vi "Autonomous Independent.vi"() -> ()   [LabVIEW 2017]
doc: "This VI is called when autonomous begins, and will automatically be terminated when autonomous ends. You can carry out timed or sensor driven robot movement independently without needing to return to the caller."
uses:
  Public/Documents/Cross The Road Electronics/Phoenix-LabVIEW/Motor Controller/Controls/CTRE_Phoenix_MotorControl_FeedbackDevice.ctl
  <vilib>/Rock Robotics/WPI/Solenoid/WPI_SolenoidValue.ctl
  Public/Documents/Cross The Road Electronics/Phoenix-LabVIEW/Motor Controller/Controls/CTRE_Phoenix_MotorControl_ControlMode.ctl
  <vilib>/Rock Robotics/WPI/Utilities/WPI_GetSetVariantRefNum.vi
  <vilib>/Rock Robotics/Network Tables/NT Read String.vi
  <vilib>/Rock Robotics/Network Tables/NT Write Numeric Array.vi
  <vilib>/Rock Robotics/WPI/Solenoid/WPI_SolenoidSetEnum.vi
  Public/Documents/Cross The Road Electronics/Phoenix-LabVIEW/Motor Controller/Get/CTRE_Phoenix_MotorController_GetSelectedSensorData.vi
  <vilib>/addons/control/pid/pid.llb/PID (DBL).vi
  Public/Documents/Cross The Road Electronics/Phoenix-LabVIEW/Motor Controller/Get/CTRE_Phoenix_MotorController_GetLimitSwitchStates.vi
  FIRST-3958-Controls-Library/NavX/navX Library v2/navX Library v2.lvlib
  <vilib>/addons/control/pid/NI_PID_pid.lvlib
panel:
  in  "Array":T1(array[cluster])=[{"Type"="Drive", "Parameter 1"=2.0, "Parameter 2"=0.0, "Parameter 3"=0.0, "Parameter 4"=0.5, "Field Angle"=FALSE}, {"Type"="Drive", "Parameter 1"=5.0, "Parameter 2"=45.0, "Parameter 3"=0.0, "Parameter 4"=0.6, "Field Angle"=TRUE}, {"Type"="Drive", "Parameter 1"=10.0, "Parameter 2"=0.0, "Parameter 3"=1.6, "Parameter 4"=0.5, "Field Angle"=FALSE}, {"Type"="Lift", "Parameter 1"=-1000.0, "Parameter 2"=0.0, "Parameter 3"=0.3, "Parameter 4"=0.5, "Field Angle"=FALSE}, {"Type"="Wait", "Parameter 1"=0.5, "Parameter 2"=0.0, "Parameter 3"=0.0, "Parameter 4"=0.0, "Field Angle"=FALSE}, {"Type"="Drive", "Parameter 1"=-4.3, "Parameter 2"=0.0, "Parameter 3"=0.0, "Parameter 4"=0.5, "Field Angle"=FALSE}, {"Type"="Turn", "Parameter 1"=0.0, "Parameter 2"=-90.0, "Parameter 3"=0.0, "Parameter 4"=0.5, "Field Angle"=TRUE}, {"Type"="Drive", "Parameter 1"=4.0, "Parameter 2"=-90.0, "Parameter 3"=0.0, "Parameter 4"=0.3, "Field Angle"=TRUE}, {"Type"="Turn", "Parameter 1"=0.0, "Parameter 2"=0.0, "Parameter 3"=0.0, "Parameter 4"=0.5, "Field Angle"=FALSE}, {"Type"="Lift", "Parameter 1"=-2170.0, "Parameter 2"=0.0, "Parameter 3"=1.5, "Parameter 4"=0.5, "Field Angle"=FALSE}, {"Type"="Intake", "Parameter 1"=1.0, "Parameter 2"=0.0, "Parameter 3"=0.0, "Parameter 4"=0.0, "Field Angle"=FALSE}, {"Type"="Grab", "Parameter 1"=1.0, "Parameter 2"=0.0, "Parameter 3"=0.0, "Parameter 4"=0.0, "Field Angle"=FALSE}, {"Type"="Drive", "Parameter 1"=3.0, "Parameter 2"=0.0, "Parameter 3"=0.5, "Parameter 4"=0.5, "Field Angle"=FALSE}, {"Type"="Grab", "Parameter 1"=0.0, "Parameter 2"=0.0, "Parameter 3"=0.0, "Parameter 4"=0.0, "Field Angle"=FALSE}, {"Type"="Intake", "Parameter 1"=0.0, "Parameter 2"=0.0, "Parameter 3"=0.0, "Parameter 4"=0.0, "Field Angle"=FALSE}, {"Type"="Drive", "Parameter 1"=-3.0, "Parameter 2"=0.0, "Parameter 3"=0.0, "Parameter 4"=0.5, "Field Angle"=FALSE}, {"Type"="Turn", "Parameter 1"=0.0, "Parameter 2"=90.0, "Parameter 3"=0.0, "Parameter 4"=0.5, "Field Angle"=TRUE}, {"Type"="Drive", "Parameter 1"=4.6, "Parameter 2"=90.0, "Parameter 3"=0.0, "Parameter 4"=0.6, "Field Angle"=TRUE}, {"Type"="Turn", "Parameter 1"=0.0, "Parameter 2"=0.0, "Parameter 3"=0.0, "Parameter 4"=0.5, "Field Angle"=FALSE}, {"Type"="Drive", "Parameter 1"=10.0, "Parameter 2"=0.0, "Parameter 3"=0.0, "Parameter 4"=0.6, "Field Angle"=FALSE}, {"Type"="Lift", "Parameter 1"=0.0, "Parameter 2"=0.0, "Parameter 3"=1.5, "Parameter 4"=0.5, "Field Angle"=FALSE}, {"Type"="Intake", "Parameter 1"=-1.0, "Parameter 2"=0.0, "Parameter 3"=0.0, "Parameter 4"=0.0, "Field Angle"=FALSE}]
  in  "stop":bool
  in  "elevator PID":T2={"proportional gain (Kc)"=0.005, "integral time (Ti, min)"=0.0, "derivative time (Td, min)"=0.0} {"derivative time (Td, min)" format="%.3f"; "integral time (Ti, min)" format="%.3f"; "proportional gain (Kc)" format="%.3f"}
  in  "elevatorPosition":dbl=1500.0 format="%.2f"
  in  "forward PID":T2={"proportional gain (Kc)"=0.001, "integral time (Ti, min)"=0.0, "derivative time (Td, min)"=0.0} {"derivative time (Td, min)" format="%.3f"; "integral time (Ti, min)" format="%.3f"; "proportional gain (Kc)" format="%.3f"}
  in  "angle PID":T2={"proportional gain (Kc)"=0.018, "integral time (Ti, min)"=0.0, "derivative time (Td, min)"=0.0} {"derivative time (Td, min)" format="%.3f"; "integral time (Ti, min)" format="%.3f"; "proportional gain (Kc)" format="%.3f"}
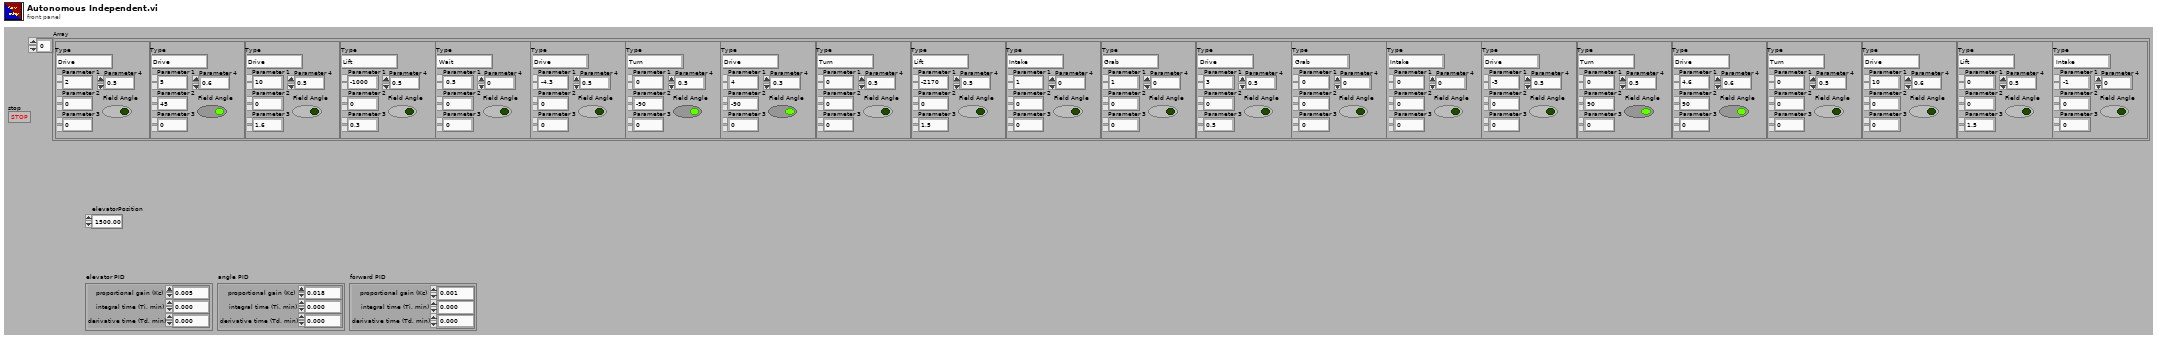
[diagram p1: front panel]
types:
  T1 = cluster{"Type":string, "Parameter 1":dbl, "Parameter 2":dbl, "Parameter 3":dbl, "Parameter 4":dbl, "Field Angle":bool}[]
  T2 = cluster{"proportional gain (Kc)":dbl, "integral time (Ti, min)":dbl, "derivative time (Td, min)":dbl}
  T3 = typedef "WPI_SolenoidValue.ctl" = enum16{"Off", "On", "Forward", "Reverse"}
  T4 = typedef "CTRE_Phoenix_MotorControl_FeedbackDevice.ctl" = i8
  T5 = typedef "WPI_JoystickDevRef.ctl" = cluster{"Device":T6}
  T6 = typedef "WPI_JoystickDeviceEnum.ctl" = enum16{"USB 0", "USB 1", "USB 2", "USB 3", "USB 4", "USB 5"}
  T7 = typedef "WPI_MotorControlDeviceRef.ctl" = cluster{"DeviceStatus":errorcluster, "Type":T8, "PWM":cluster{"PWM Channel":T9, "DeadBand":T10}, "CAN":cluster{"Device Number":u8, "SetOutput VI Ref":variant, "GetOutput VI Ref":variant, "Enable VI Ref":variant, "Disable VI Ref":variant, "Data":variant}, "Invert":bool, "DIO PWM":cluster{"PWM \"Enable\" Channel":T9, "DIOChannel":T11, "PWM Rate":dbl}}
  T8 = typedef "WPI_MotorControlType.ctl" = enum16{"PWM", "CAN", "DIO PWM"}
  T9 = typedef "FPGA_DIOPWMChannel.ctl" = enum8{"PWM 0", "PWM 1", "PWM 2", "PWM 3", "PWM 4", "PWM 5", "PWM 6", "PWM 7", "PWM 8", "PWM 9", "PWM MXP 0", "PWM MXP 1", "PWM MXP 2", "PWM MXP 3", "PWM MXP 4", "PWM MXP 5", "PWM MXP 6", "PWM MXP 7", "PWM MXP 8", "PWM MXP 9", "Invalid"}
  T10 = typedef "WPI_PWMDeadband.ctl" = cluster{"Name":string, "maxPositivePwm":i32, "minPositivePwm":i32, "centerPwm":i32, "maxNegativePwm":i32, "minNegativePwm":i32, "angularRange":u16}
  T11 = typedef "FPGA_DIOChannel.ctl" = enum8{"DIO 0", "DIO 1", "DIO 2", "DIO 3", "DIO 4", "DIO 5", "DIO 6", "DIO 7", "DIO 8", "DIO 9", "DIO MXP 0", "DIO MXP 1", "DIO MXP 2", "DIO MXP 3", "DIO MXP 4", "DIO MXP 5", "DIO MXP 6", "DIO MXP 7", "DIO MXP 8", "DIO MXP 9", "DIO MXP 10", "DIO MXP 11", "DIO MXP 12", "DIO MXP 13", "DIO MXP 14", "DIO MXP 15", "SPI Port CS1", "SPI Port CS2", "SPI Port CS3", "SPI Port MISO", "SPI Port MOSI", "Invalid"}
  T12 = typedef "WPI_SolenoidDevRef.ctl" = cluster{"DevStatus":errorcluster, "Pneumatics Control Module":u8, "Forward Solenoid Channel":T13, "Reverse Solenoid Channel":T13}
  T13 = typedef "WPI_SolenoidChannel.ctl" = enum8{"Solenoid 0", "Solenoid 1", "Solenoid 2", "Solenoid 3", "Solenoid 4", "Solenoid 5", "Solenoid 6", "Solenoid 7", "Invalid"}
  T14 = typedef "navX Library v2.lvlib/Z900_navX_DeviceTypeDef.ctl" = cluster{"Interface":cluster{"Protocol":T15, "Update Rate (4Hz-100Hz)":u8, "navX Open TypeDef":variant}, "Notify Packet":refnum<notifier>, "Loop VI Refnum":refnum<vi>, "Ready to Close Occurrence Refnum":refnum<k4>}
  T15 = typedef "navX Library v2.lvlib/Z900_navX_ProtocolTypeDef.ctl" = enum16{"SERIAL", "I2C", "SPI"}
  T16 = typedef "CTRE_Phoenix_MotorControl_ControlMode.ctl" = u16
  T17 = cluster{"Yaw":dbl, "Roll":dbl, "Pitch":dbl, "Heading":dbl, "Fused Heading":dbl}
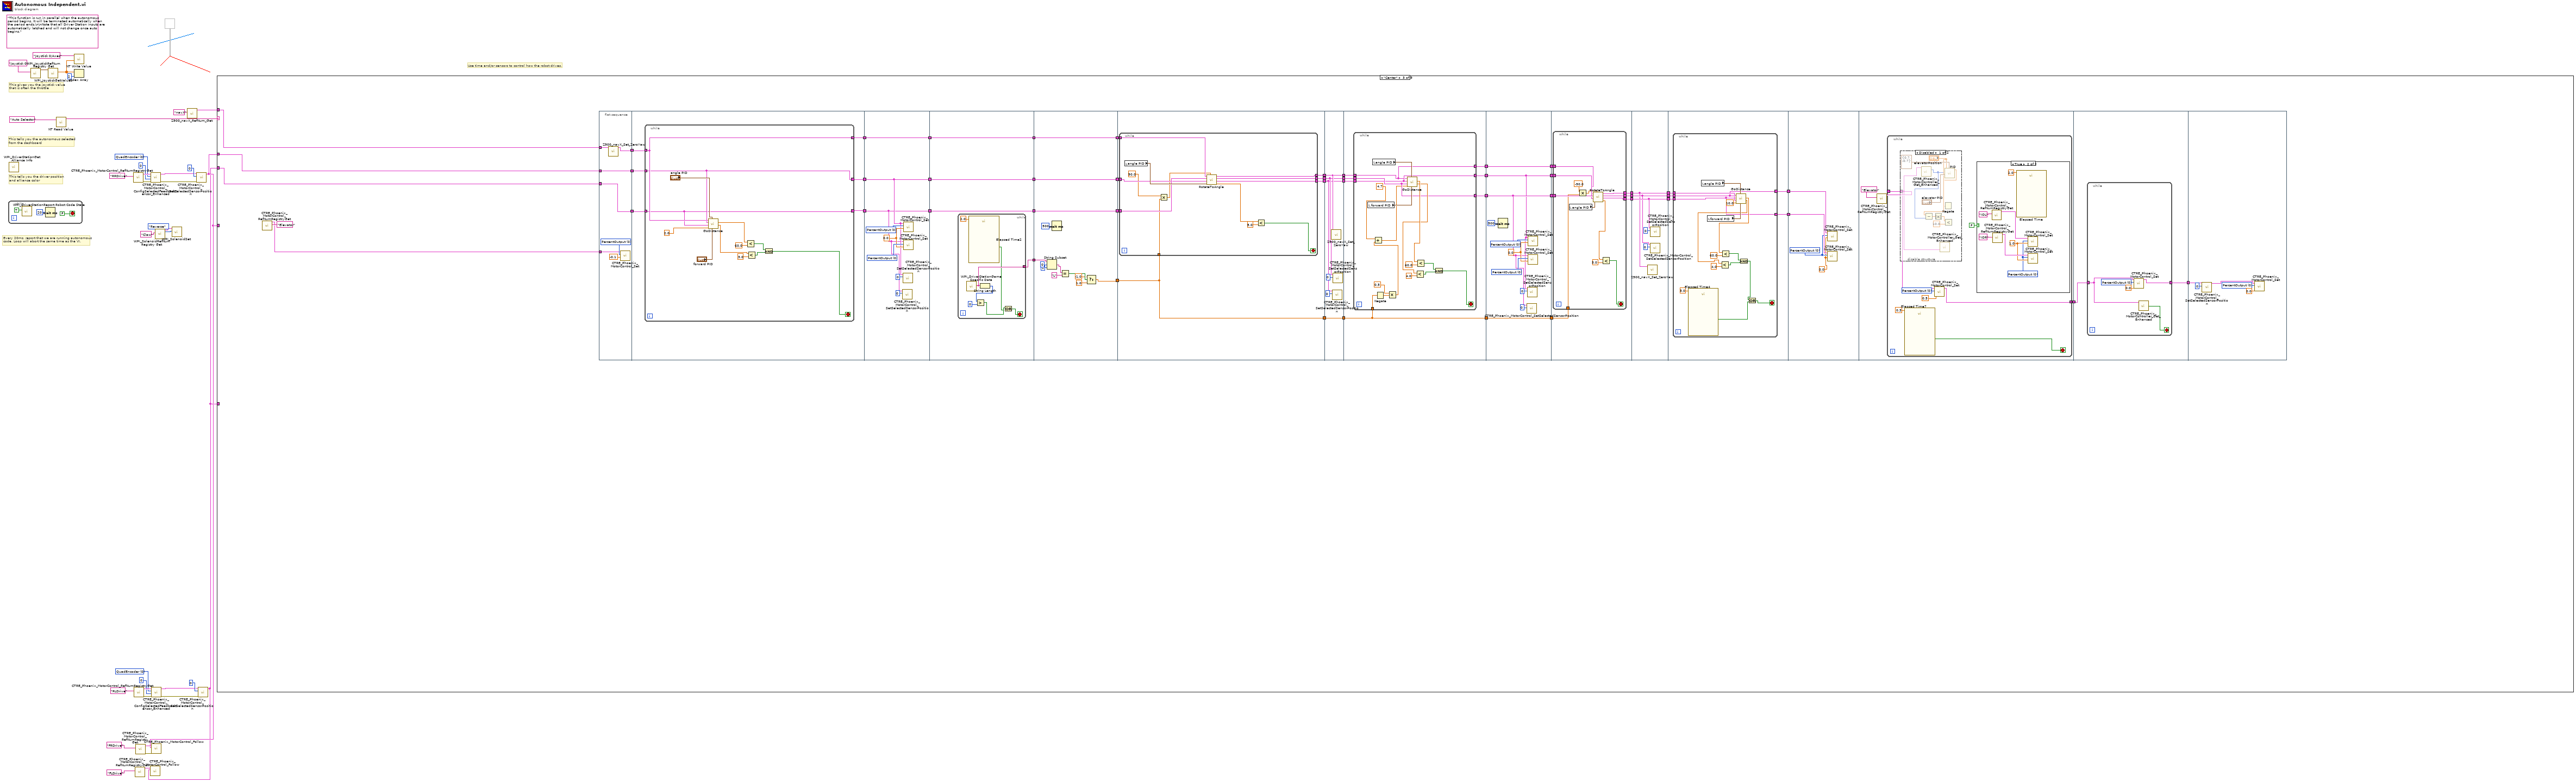
[diagram p0: block diagram]
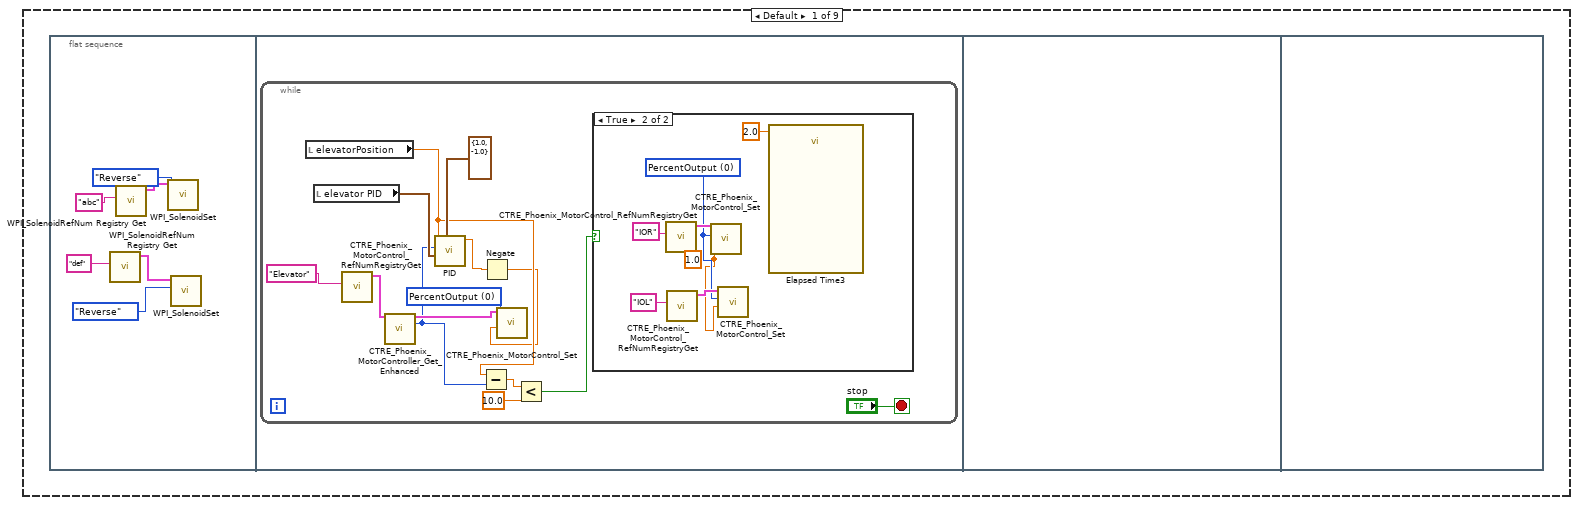
[diagram p2: hidden frame]
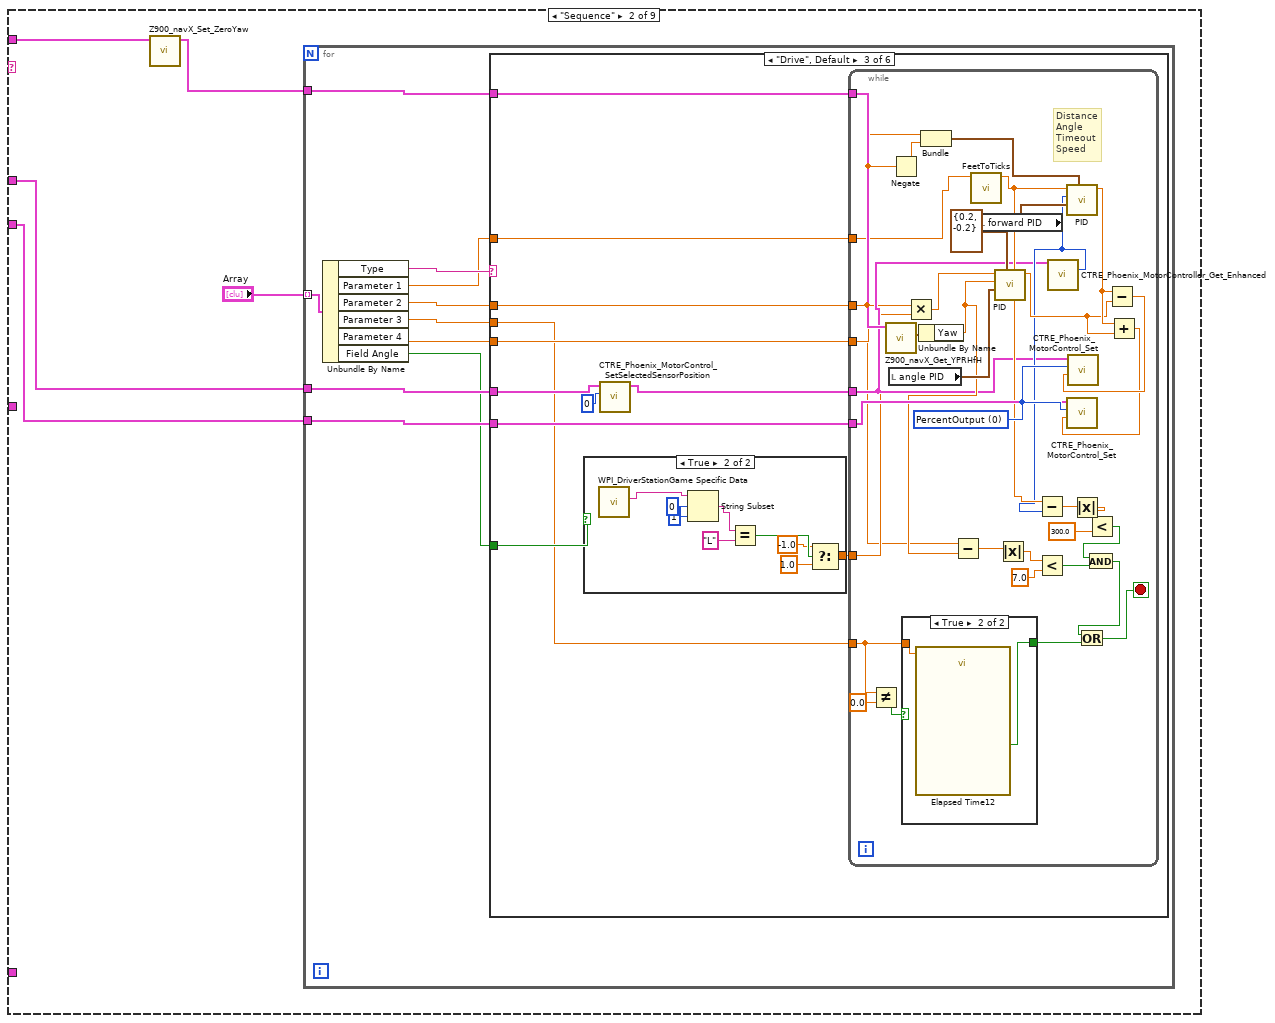
[diagram p4: hidden frame]
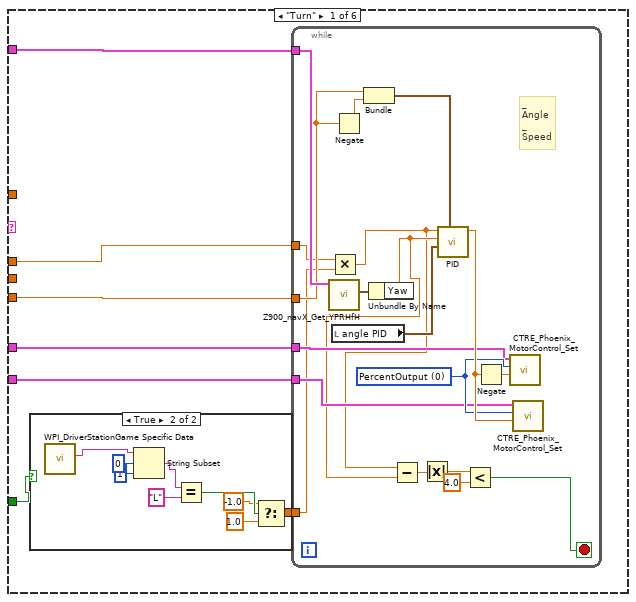
[diagram p5: hidden frame]
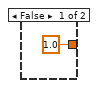
[diagram p6: hidden frame]
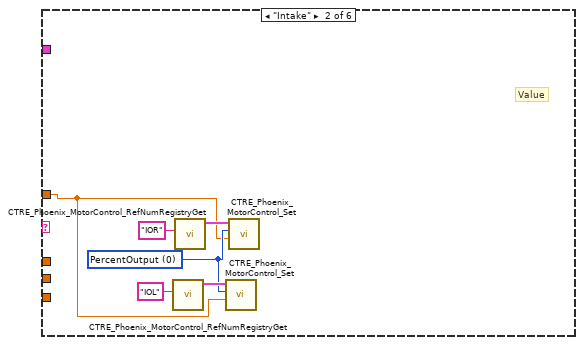
[diagram p7: hidden frame]
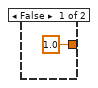
[diagram p8: hidden frame]
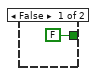
[diagram p9: hidden frame]
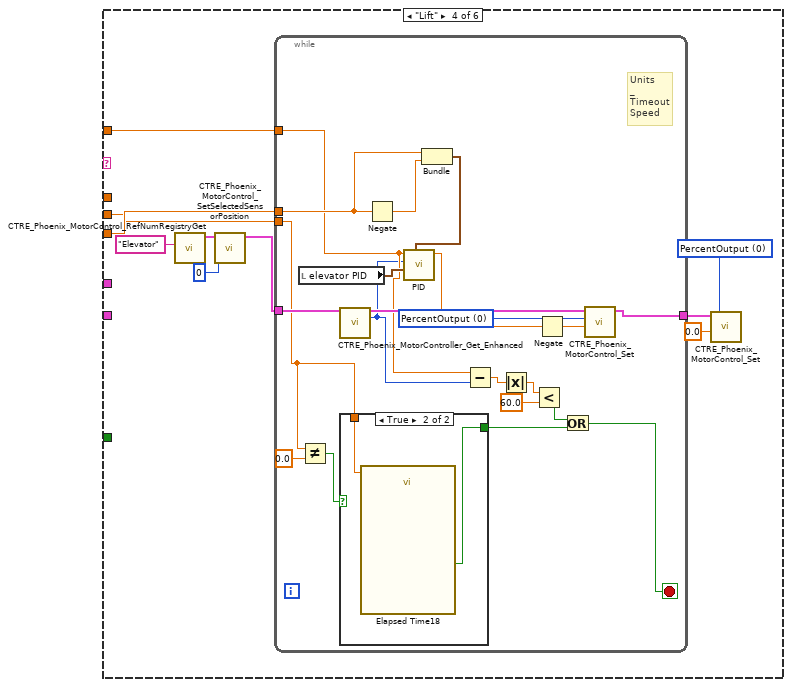
[diagram p10: hidden frame]
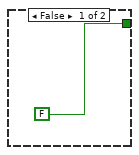
[diagram p11: hidden frame]
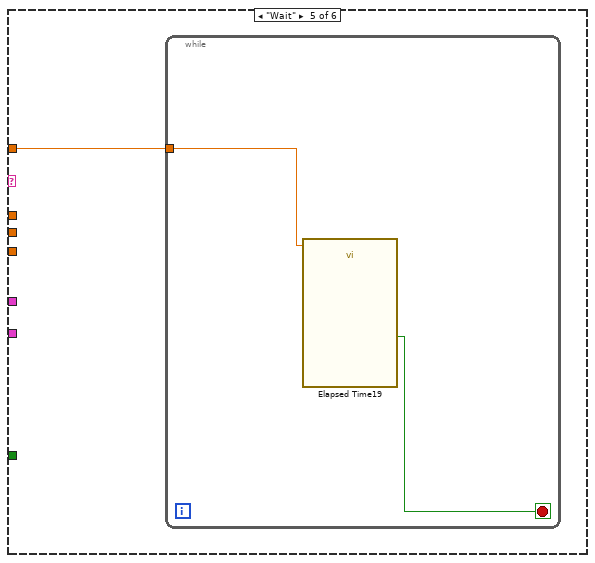
[diagram p12: hidden frame]
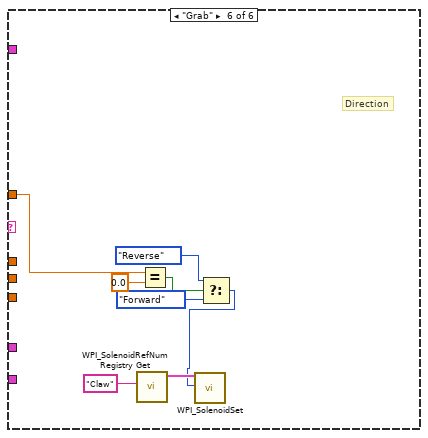
[diagram p13: hidden frame]
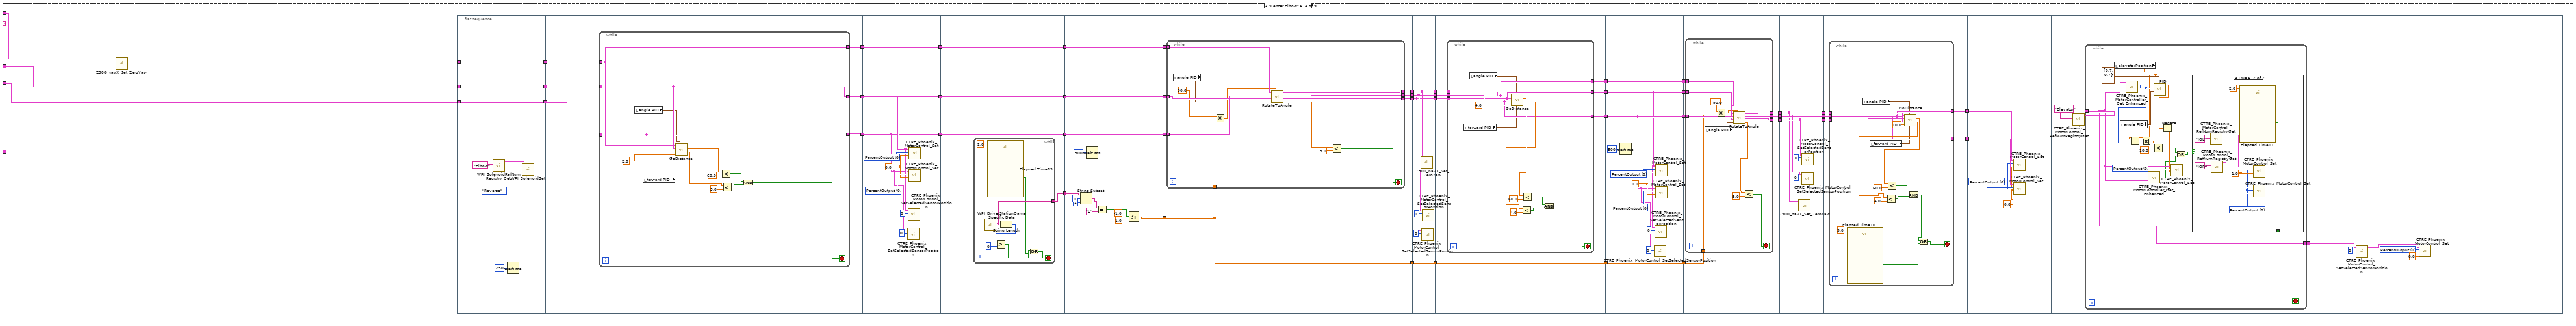
[diagram p16: hidden frame]
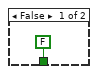
[diagram p17: hidden frame]
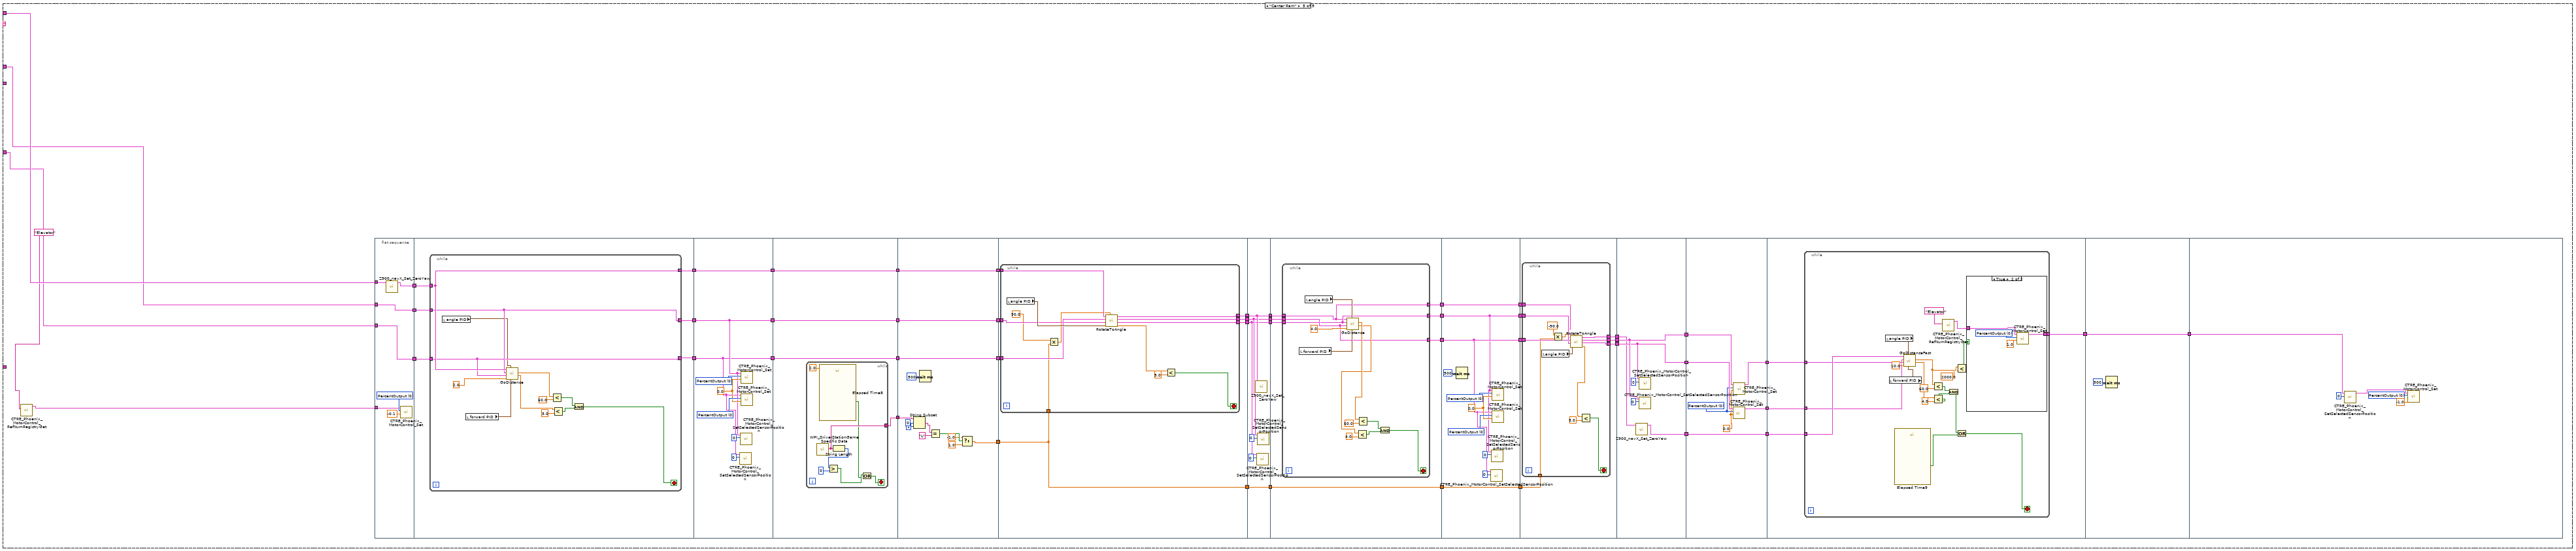
[diagram p18: hidden frame]
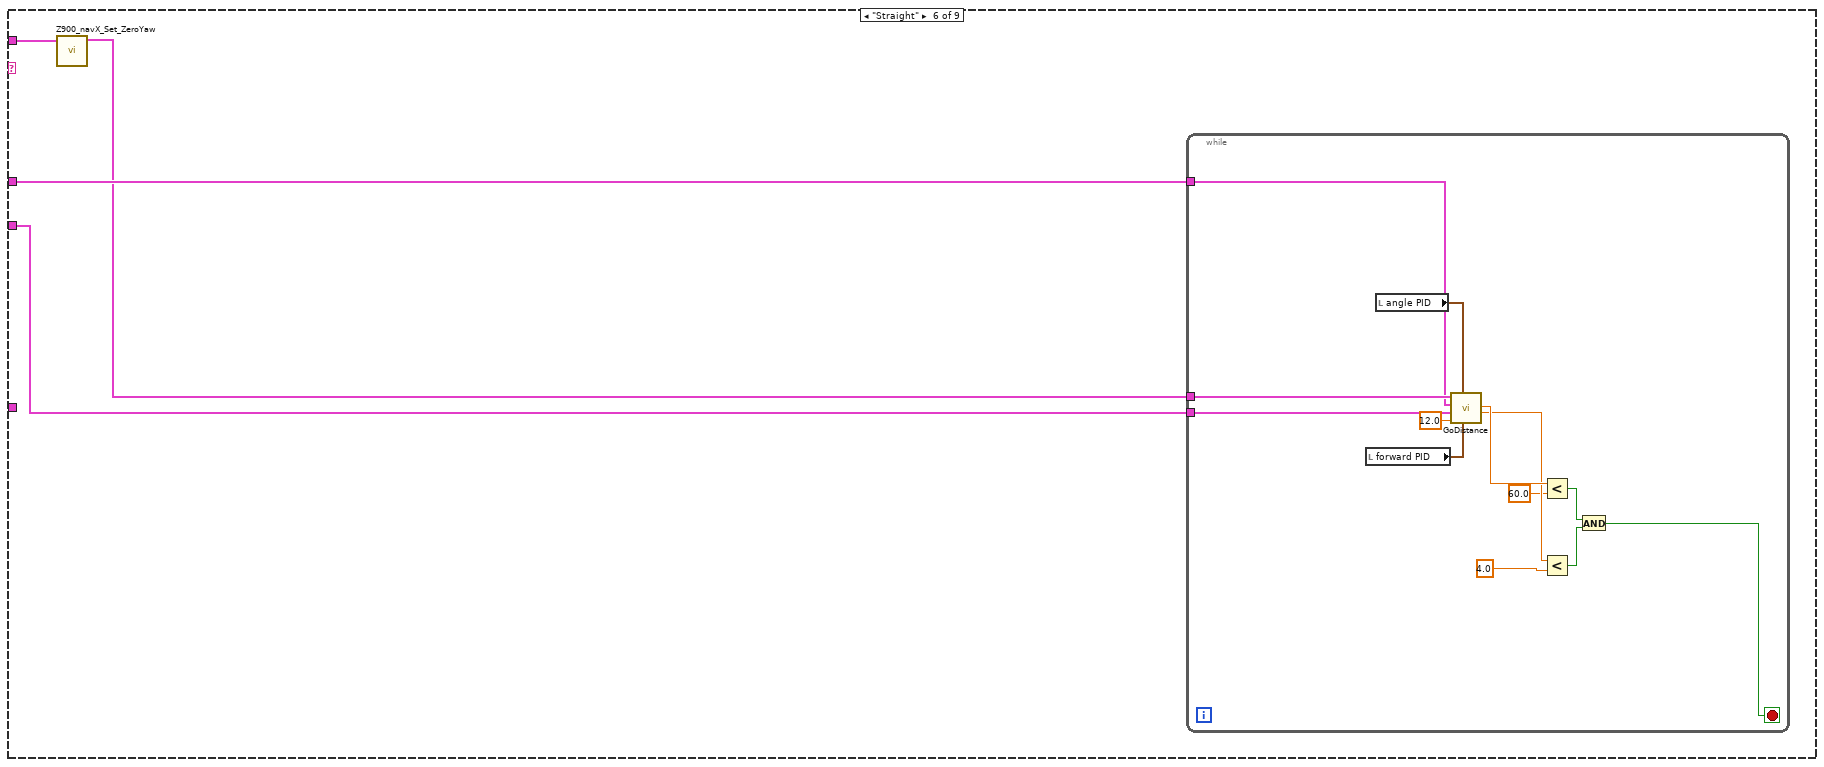
[diagram p20: hidden frame]
diagram:
  w19 = T4 0 items=["None"=-1, "QuadEncoder"=0, "Analog"=2, "Tachometer"=4, "Pulse Width Encoded Position"=8, "Sensor Sum (S0 + S1)"=9, "Sensor Difference (D0 - D1)"=10, "Remote Source 0"=11, "Remote Source 1"=12, "Software Emulated"=15] ("Feedback Device")
  w24 = T4 0 items=["None"=-1, "QuadEncoder"=0, "Analog"=2, "Tachometer"=4, "Pulse Width Encoded Position"=8, "Sensor Sum (S0 + S1)"=9, "Sensor Difference (D0 - D1)"=10, "Remote Source 0"=11, "Remote Source 1"=12, "Software Emulated"=15] ("Feedback Device")
  (unwired) "This function is run in parallel when the autonomous period begins. It will be terminated automatically when the period ends.\n\nNote that all Driver Station inputs are automatically latched and will not change once auto begins."
  # "This tells you the autonomous selected\nfrom the dashboard"
  # "Every 20ms, report that we are running autonomous\ncode. Loop will abort the same time as the VI."
  # "This gives you the joystick value\nthat is often the throttle"
  # "Use time and/or sensors to control how the robot drives."
  # "This tells you the driver position\nand alliance color"
  n1 = while {
    stop <- FALSE stop-if-true
    n2 = call <vilib>:"WPI_DriverStationReport Robot Code State.vi"("Autonomous"=TRUE) -> ()  [unwired: 10 in, 1 out]
    n3 = Wait (ms)(milliseconds to wait=u32 20) -> ()  [unwired: 1 out]
  }
  n4 = call <vilib>:"WPI_DriverStationGet Alliance Info.vi"() -> ()  [unwired: 12 out]
  n5 = call <vilib>:"WPI_JoystickRefNum Registry Get.vi"("refnum name"="Joystick 0") -> ("JoystickDevRef"=w34:T5)  [unwired: 1 in, 9 out]
  n6 = call <vilib>:"WPI_JoystickGetValues.vi"("JoystickDevRef"=w34) -> ("Axes"=w30:dbl[])  [unwired: 6 in, 4 out]
  n7 = call-poly <vilib>:"NT Read Value.vi"("Name"="Auto Selector") -> ("String"=w31:string)  [unwired: 9 in, 1 out]
  n8 = call-poly <vilib>:"NT Write Value.vi"("Numeric Array"=w30, "Name"="Joystick 0/Axes") -> ()  [unwired: 9 in, 1 out]
  n9 = Index Array(array=w30, index=2) -> ()  [unwired: 1 out]
  n10 = call "CTRE_Phoenix_MotorControl_RefNumRegistryGet.vi"("refnum name"="RRDrive") -> ("error out"=w27:errorcluster, "PhoenixMotorControlDevRef"=w26:T7)  [unwired: 9 in]
  n11 = call "CTRE_Phoenix_MotorControl_RefNumRegistryGet.vi"("refnum name"="RLDrive") -> ("error out"=w22:errorcluster, "PhoenixMotorControlDevRef"=w21:T7)  [unwired: 9 in]
  n12 = call "CTRE_Phoenix_MotorControl_RefNumRegistryGet.vi"("refnum name"="FLDrive") -> ("PhoenixMotorControlDevRef"=w10:T7)  [unwired: 9 in, 1 out]
  n13 = call "CTRE_Phoenix_MotorControl_RefNumRegistryGet.vi"("refnum name"="FRDrive") -> ("error out"=w12:errorcluster, "PhoenixMotorControlDevRef"=w11:T7)  [unwired: 9 in]
  n14 = call "CTRE_Phoenix_MotorControl_ConfigSelectedFeedbackSensor_Enhanced.vi"("error in (no error)"=w27, "pidLoopIdx"=0, "Feedback Device"=w24, "PhoenixMotorControlDevRef"=w26) -> ("error out"=w6:errorcluster, "PhoenixMotorControlDevRef"=w7:T7)  [unwired: 6 in]
  n15 = call "CTRE_Phoenix_MotorControl_ConfigSelectedFeedbackSensor_Enhanced.vi"("error in (no error)"=w22, "pidLoopIdx"=0, "Feedback Device"=w19, "PhoenixMotorControlDevRef"=w21) -> ("error out"=w4:errorcluster, "PhoenixMotorControlDevRef"=w5:T7)  [unwired: 6 in]
  n16 = call <vilib>:"WPI_SolenoidRefNum Registry Get.vi"("refnum name"="Claw") -> ("SolenoidDevRef"=w3:T12)  [unwired: 9 in, 1 out]
  n17 = call-poly <vilib>:"WPI_SolenoidSet.vi"("Value"=WPI_SolenoidValue."Reverse", "SolenoidDevRef"=w3) -> ()  [unwired: 8 in, 2 out]
  n18 = call "Z900_navX_RefNum_Get.vi"("refnum name"="navX") -> ("navX Device"=w15:T14)  [unwired: 9 in, 1 out]
  n19 = call "CTRE_Phoenix_MotorControl_SetSelectedSensorPosition.vi"("error in (no error)"=w6, "New Sensor Position"=0, "PhoenixMotorControlDevRef"=w7) -> ("PhoenixMotorControlDevRef"=w9:T7)  [unwired: 7 in, 1 out]
  n20 = call "CTRE_Phoenix_MotorControl_Follow.vi"("error in (no error)"=w12, "Master Controller to Follow"=w9, "PhoenixMotorControlDevRef"=w11) -> ()  [unwired: 7 in, 2 out]
  n21 = call "CTRE_Phoenix_MotorControl_SetSelectedSensorPosition.vi"("error in (no error)"=w4, "New Sensor Position"=0, "PhoenixMotorControlDevRef"=w5) -> ("PhoenixMotorControlDevRef"=w8:T7)  [unwired: 7 in, 1 out]
  n22 = call "CTRE_Phoenix_MotorControl_Follow.vi"("Master Controller to Follow"=w8, "PhoenixMotorControlDevRef"=w10) -> ()  [unwired: 8 in, 2 out]
  n23 = case shown="\"Center\"" w31 {
    tunnel: w9 -> [_ w67 w272 w528 w734 w959 w975 w1069 _]
    tunnel: w8 -> [_ w66 w271 w527 _ w960 w974 w1068 _]
    tunnel: w15 -> [_ w69 w275 w487 w735 w958 w976 w1070 _]
    tunnel: w9 -> [_ _ _ _ w733 _ _ _ _]
    tunnel: w8 -> [_ _ _ _ _ _ _ _ _]
    frame Default {
      n24 = flat-sequence {
        frame #0 {
          n25 = call <vilib>:"WPI_SolenoidRefNum Registry Get.vi"("refnum name"="def") -> ("SolenoidDevRef"=w42:T12)  [unwired: 9 in, 1 out]
          n26 = call <vilib>:"WPI_SolenoidRefNum Registry Get.vi"("refnum name"="abc") -> ("SolenoidDevRef"=w41:T12)  [unwired: 9 in, 1 out]
          n27 = call-poly <vilib>:"WPI_SolenoidSet.vi"("Value"=WPI_SolenoidValue."Reverse", "SolenoidDevRef"=w41) -> ()  [unwired: 8 in, 2 out]
          n28 = call-poly <vilib>:"WPI_SolenoidSet.vi"("Value"=WPI_SolenoidValue."Reverse", "SolenoidDevRef"=w42) -> ()  [unwired: 8 in, 2 out]
        }
        frame #1 {
          n29 = while {
            stop <- "stop" stop-if-true
            w54 = T16 0 items=["PercentOutput"=0, "Position"=1, "Velocity"=2, "Current"=3, "Follower"=5, "MotionProfile"=6, "MotionMagic"=7, "MotionMagicArc"=8, "MotionProfileArc"=10, "Disabled"=15] ("Control Mode")
            n30 = local read "elevatorPosition"() -> (w52:dbl)
            n31 = local read "elevator PID"() -> (w58:T2)
            n32 = call "CTRE_Phoenix_MotorControl_RefNumRegistryGet.vi"("refnum name"="Elevator") -> ("PhoenixMotorControlDevRef"=w56:T7)  [unwired: 9 in, 1 out]
            n33 = call-poly "CTRE_Phoenix_MotorController_Get_Enhanced.vi"("PhoenixMotorControlDevRef"=w56) -> ("PhoenixMotorControlDevRef"=w53:T7, "Position (Raw Sensor Units)"=w51:i32)  [unwired: 11 in, 2 out]
            n34 = call-poly <vilib>:"PID.vi"("output range"=cluster{"output high":dbl, "output low":dbl} {"output high"=1.0, "output low"=-1.0}, "PID gains"=w58, "process variable"=w51, "setpoint"=w52) -> ("output"=w48:dbl)  [unwired: 6 in, 1 out]
            n35 = Subtract(x=w52, y=w51) -> (x-y=w50:dbl)
            n36 = Negate(x=w48) -> (-x=w47:dbl)
            n37 = call "CTRE_Phoenix_MotorControl_Set.vi"("Output"=w47, "Control Mode"=w54, "PhoenixMotorControlDevRef"=w53) -> ()  [unwired: 7 in, 2 out]
            n38 = Less?(x=w50, y=10.0) -> (x < y?=w45:bool)
            n39 = case shown="True" w45 {
              frame False {
              }
              frame True {
                w60 = 1.0 ("Output")
                w61 = T16 0 items=["PercentOutput"=0, "Position"=1, "Velocity"=2, "Current"=3, "Follower"=5, "MotionProfile"=6, "MotionMagic"=7, "MotionMagicArc"=8, "MotionProfileArc"=10, "Disabled"=15] ("Control Mode")
                n40 = call "CTRE_Phoenix_MotorControl_RefNumRegistryGet.vi"("refnum name"="IOR") -> ("PhoenixMotorControlDevRef"=w62:T7)  [unwired: 9 in, 1 out]
                n41 = call "CTRE_Phoenix_MotorControl_RefNumRegistryGet.vi"("refnum name"="IOL") -> ("PhoenixMotorControlDevRef"=w63:T7)  [unwired: 9 in, 1 out]
                n42 = call "CTRE_Phoenix_MotorControl_Set.vi"("Output"=w60, "Control Mode"=w61, "PhoenixMotorControlDevRef"=w62) -> ()  [unwired: 7 in, 2 out]
                n43 = call "CTRE_Phoenix_MotorControl_Set.vi"("Output"=w60, "Control Mode"=w61, "PhoenixMotorControlDevRef"=w63) -> ()  [unwired: 7 in, 2 out]
                n44 = call "Elapsed Time3"("Time Target (s)"=2.0) -> ()  [unwired: 11 in, 8 out]
              }
            }
          }
        }
        frame #2 {
        }
        frame #3 {
        }
      }
    }
    frame "Sequence" {
      n45 = call "Z900_navX_Set_ZeroYaw.vi"("navX Device"=w69) -> ("navX Device"=w68:T14)  [unwired: 9 in, 1 out]
      n46 = for {
        tunnel: "Array" -> [w80] mode=indexing
        tunnel: w68 -> [w78]
        tunnel: w67 -> [w74]
        tunnel: w66 -> [w73]
        n47 = Unbundle By Name(w80) -> ("Type"=w79:string, "Parameter 1"=w75:dbl, "Parameter 2"=w76:dbl, "Parameter 3"=w71:dbl, "Parameter 4"=w77:dbl, "Field Angle"=w72:bool)
        n48 = case shown="\"Drive\", Default" w79 {
          tunnel: w77 -> [w85 _ w132 w188 _ _]
          tunnel: w76 -> [w87 _ w133 _ _ _]
          tunnel: w78 -> [w86 _ w131 _ _ _]
          tunnel: w75 -> [_ w117 w130 w187 w217 w227]
          tunnel: w74 -> [w84 _ w128 _ _ _]
          tunnel: w73 -> [w83 _ w129 _ _ _]
          tunnel: w72 -> [w82 _ w125 _ _ _]
          tunnel: w71 -> [_ _ w123 w186 _ _]
          frame "Turn" {
            n49 = case shown="True" w82 {
              tunnel: [1.0 ("f") w89] -> w81
              frame False {
              }
              frame True {
                n50 = call <vilib>:"WPI_DriverStationGame Specific Data.vi"() -> ("Game Specific Data"=w90:string)  [unwired: 11 in]
                n51 = String Subset(string=w90, offset (0)=0, length (rest)=1 ("length (rest)")) -> (substring=w96:string)
                n52 = Equal?(x=w96, y="L") -> (x = y?=w97:bool)
                n53 = Select(t=-1.0, s=w97, f=1.0) -> (s? t:f=w89:dbl)
              }
            }
            n54 = while {
              tunnel: w87 -> [w99]
              tunnel: w86 -> [w115]
              tunnel: w85 -> [w114]
              tunnel: w84 -> [w107]
              tunnel: w83 -> [w106]
              tunnel: w81 -> [w100]
              stop <- w101 stop-if-true
              w108 = T16 0 items=["PercentOutput"=0, "Position"=1, "Velocity"=2, "Current"=3, "Follower"=5, "MotionProfile"=6, "MotionMagic"=7, "MotionMagicArc"=8, "MotionProfileArc"=10, "Disabled"=15] ("Control Mode")
              # "_\nAngle\n_\nSpeed"
              n55 = call "Z900_navX_Get_YPRHfH.vi"("navX Device"=w115) -> ("YRPHfH"=w116:T17)  [unwired: 7 in, 3 out]
              n56 = Multiply(x=w99, y=w100) -> (x*y=w98:dbl)
              n57 = local read "angle PID"() -> (w111:T2)
              n58 = Negate(x=w114) -> (-x=w113:dbl)
              n59 = Bundle("Parameter 4"=w114, w113) -> (w112:cluster{"Parameter 4":dbl, dbl})  [unwired: 1 in]
              n60 = Unbundle By Name(w116) -> ("Yaw"=w104:dbl)
              n61 = Subtract(x=w98, y=w104) -> (x-y=w105:dbl)
              n62 = Absolute Value(x=w105) -> (abs(x)=w103:dbl)
              n63 = call-poly <vilib>:"PID.vi"("output range"=w112, "PID gains"=w111, "process variable"=w104, "setpoint"=w98) -> ("output"=w110:dbl)  [unwired: 6 in, 1 out]
              n64 = Less?(x=w103, y=4.0) -> (x < y?=w101:bool)
              n65 = Negate(x=w110) -> (-x=w109:dbl)
              n66 = call "CTRE_Phoenix_MotorControl_Set.vi"("Output"=w109, "Control Mode"=w108, "PhoenixMotorControlDevRef"=w107) -> ()  [unwired: 7 in, 2 out]
              n67 = call "CTRE_Phoenix_MotorControl_Set.vi"("Output"=w110, "Control Mode"=w108, "PhoenixMotorControlDevRef"=w106) -> ()  [unwired: 7 in, 2 out]
            }
          }
          frame "Intake" {
            w118 = T16 0 items=["PercentOutput"=0, "Position"=1, "Velocity"=2, "Current"=3, "Follower"=5, "MotionProfile"=6, "MotionMagic"=7, "MotionMagicArc"=8, "MotionProfileArc"=10, "Disabled"=15] ("Control Mode")
            # "Value"
            n68 = call "CTRE_Phoenix_MotorControl_RefNumRegistryGet.vi"("refnum name"="IOL") -> ("PhoenixMotorControlDevRef"=w119:T7)  [unwired: 9 in, 1 out]
            n69 = call "CTRE_Phoenix_MotorControl_RefNumRegistryGet.vi"("refnum name"="IOR") -> ("PhoenixMotorControlDevRef"=w120:T7)  [unwired: 9 in, 1 out]
            n70 = call "CTRE_Phoenix_MotorControl_Set.vi"("Output"=w117, "Control Mode"=w118, "PhoenixMotorControlDevRef"=w119) -> ()  [unwired: 7 in, 2 out]
            n71 = call "CTRE_Phoenix_MotorControl_Set.vi"("Output"=w117, "Control Mode"=w118, "PhoenixMotorControlDevRef"=w120) -> ()  [unwired: 7 in, 2 out]
          }
          frame "Drive", Default {
            n72 = case shown="True" w125 {
              tunnel: [1.0 ("f") w135] -> w124
              frame False {
              }
              frame True {
                n73 = call <vilib>:"WPI_DriverStationGame Specific Data.vi"() -> ("Game Specific Data"=w136:string)  [unwired: 11 in]
                n74 = String Subset(string=w136, offset (0)=0, length (rest)=1 ("length (rest)")) -> (substring=w142:string)
                n75 = Equal?(x=w142, y="L") -> (x = y?=w143:bool)
                n76 = Select(t=-1.0, s=w143, f=1.0) -> (s? t:f=w135:dbl)
              }
            }
            n77 = call "CTRE_Phoenix_MotorControl_SetSelectedSensorPosition.vi"("New Sensor Position"=0, "PhoenixMotorControlDevRef"=w128) -> ("PhoenixMotorControlDevRef"=w127:T7)  [unwired: 8 in, 1 out]
            n78 = while {
              tunnel: w133 -> [w151]
              tunnel: w131 -> [w178]
              tunnel: w132 -> [w177]
              tunnel: w130 -> [w171]
              tunnel: w127 -> [w153]
              tunnel: w129 -> [w165]
              tunnel: w124 -> [w152]
              tunnel: w123 -> [w146]
              stop <- w147 stop-if-true
              w174 = T16 0 items=["PercentOutput"=0, "Position"=1, "Velocity"=2, "Current"=3, "Follower"=5, "MotionProfile"=6, "MotionMagic"=7, "MotionMagicArc"=8, "MotionProfileArc"=10, "Disabled"=15] ("Control Mode")
              # "Distance\nAngle\nTimeout\nSpeed"
              n79 = Not Equal?(x=w146, y=0.0) -> (x != y?=w144:bool)
              n80 = call "Z900_navX_Get_YPRHfH.vi"("navX Device"=w178) -> ("YRPHfH"=w179:T17)  [unwired: 7 in, 3 out]
              n81 = local read "angle PID"() -> (w175:T2)
              n82 = Negate(x=w177) -> (-x=w176:dbl)
              n83 = case shown="True" w144 {
                tunnel: [FALSE ("Time has Elapsed") w182] -> w149
                tunnel: w146 -> [_ w181]
                frame False {
                }
                frame True {
                  n84 = call "Elapsed Time12"("Time Target (s)"=w181) -> ("Time has Elapsed"=w182:bool)  [unwired: 11 in, 7 out]
                }
              }
              n85 = Multiply(x=w151, y=w152) -> (x*y=w150:dbl)
              n86 = Unbundle By Name(w179) -> ("Yaw"=w159:dbl)
              n87 = Bundle("Parameter 4"=w177, w176) -> (w173:cluster{"Parameter 4":dbl, dbl})  [unwired: 1 in]
              n88 = Subtract(x=w151, y=w159) -> (x-y=w158:dbl)
              n89 = call "FeetToTicks.vi"("x"=w171) -> ("Numeric"=w164:dbl)  [unwired: 10 in]
              n90 = local read "forward PID"() -> (w170:T2)
              n91 = call-poly <vilib>:"PID.vi"("output range"=cluster{"output high":dbl, "output low":dbl} {"output high"=0.2, "output low"=-0.2}, "PID gains"=w175, "process variable"=w159, "setpoint"=w150) -> ("output"=w168:dbl)  [unwired: 6 in, 1 out]
              n92 = Absolute Value(x=w158) -> (abs(x)=w157:dbl)
              n93 = Less?(x=w157, y=7.0) -> (x < y?=w155:bool)
              n94 = call-poly "CTRE_Phoenix_MotorController_Get_Enhanced.vi"("PhoenixMotorControlDevRef"=w153) -> ("Position (Raw Sensor Units)"=w163:i32)  [unwired: 11 in, 3 out]
              n95 = Subtract(x=w164, y=w163) -> (x-y=w162:dbl)
              n96 = call-poly <vilib>:"PID.vi"("output range"=w173, "PID gains"=w170, "process variable"=w163, "setpoint"=w164) -> ("output"=w169:dbl)  [unwired: 6 in, 1 out]
              n97 = Absolute Value(x=w162) -> (abs(x)=w161:dbl)
              n98 = Less?(x=w161, y=300.0) -> (x < y?=w154:bool)
              n99 = And(x=w154, y=w155) -> (x .and. y?=w148:bool)
              n100 = Or(x=w148, y=w149) -> (x .or. y?=w147:bool)
              n101 = Subtract(x=w169, y=w168) -> (x-y=w167:dbl)
              n102 = call "CTRE_Phoenix_MotorControl_Set.vi"("Output"=w167, "Control Mode"=w174, "PhoenixMotorControlDevRef"=w153) -> ()  [unwired: 7 in, 2 out]
              n103 = Add(x=w169, y=w168) -> (x+y=w166:dbl)
              n104 = call "CTRE_Phoenix_MotorControl_Set.vi"("Output"=w166, "Control Mode"=w174, "PhoenixMotorControlDevRef"=w165) -> ()  [unwired: 7 in, 2 out]
            }
          }
          frame "Lift" {
            w183 = T16 0 items=["PercentOutput"=0, "Position"=1, "Velocity"=2, "Current"=3, "Follower"=5, "MotionProfile"=6, "MotionMagic"=7, "MotionMagicArc"=8, "MotionProfileArc"=10, "Disabled"=15] ("Control Mode")
            n105 = call "CTRE_Phoenix_MotorControl_RefNumRegistryGet.vi"("refnum name"="Elevator") -> ("PhoenixMotorControlDevRef"=w191:T7)  [unwired: 9 in, 1 out]
            n106 = call "CTRE_Phoenix_MotorControl_SetSelectedSensorPosition.vi"("New Sensor Position"=0, "PhoenixMotorControlDevRef"=w191) -> ("PhoenixMotorControlDevRef"=w190:T7)  [unwired: 8 in, 1 out]
            n107 = while {
              tunnel: w190 -> [w213]
              tunnel: w188 -> [w211]
              tunnel: w187 -> [w205]
              tunnel: w186 -> [w198]
              tunnel: [w193] -> w184
              stop <- w195 stop-if-true
              w206 = T16 0 items=["PercentOutput"=0, "Position"=1, "Velocity"=2, "Current"=3, "Follower"=5, "MotionProfile"=6, "MotionMagic"=7, "MotionMagicArc"=8, "MotionProfileArc"=10, "Disabled"=15] ("Control Mode")
              # "Units\n_\nTimeout\nSpeed"
              n108 = local read "elevator PID"() -> (w208:T2)
              n109 = Not Equal?(x=w198, y=0.0) -> (x != y?=w197:bool)
              n110 = call-poly "CTRE_Phoenix_MotorController_Get_Enhanced.vi"("PhoenixMotorControlDevRef"=w213) -> ("PhoenixMotorControlDevRef"=w209:T7, "Position (Raw Sensor Units)"=w204:i32)  [unwired: 11 in, 2 out]
              n111 = case shown="True" w197 {
                tunnel: w198 -> [_ w216]
                tunnel: [FALSE ("Time has Elapsed") w215] -> w196
                frame False {
                }
                frame True {
                  n112 = call "Elapsed Time18"("Time Target (s)"=w216) -> ("Time has Elapsed"=w215:bool)  [unwired: 11 in, 7 out]
                }
              }
              n113 = Negate(x=w211) -> (-x=w212:dbl)
              n114 = Bundle("Parameter 4"=w211, w212) -> (w210:cluster{"Parameter 4":dbl, dbl})  [unwired: 1 in]
              n115 = call-poly <vilib>:"PID.vi"("output range"=w210, "PID gains"=w208, "process variable"=w204, "setpoint"=w205) -> ("output"=w207:dbl)  [unwired: 6 in, 1 out]
              n116 = Subtract(x=w205, y=w204) -> (x-y=w203:dbl)
              n117 = Absolute Value(x=w203) -> (abs(x)=w202:dbl)
              n118 = Less?(x=w202, y=60.0) -> (x < y?=w200:bool)
              n119 = Negate(x=w207) -> (-x=w194:dbl)
              n120 = Or(x=w200, y=w196) -> (x .or. y?=w195:bool)
              n121 = call "CTRE_Phoenix_MotorControl_Set.vi"("Output"=w194, "Control Mode"=w206, "PhoenixMotorControlDevRef"=w209) -> ("PhoenixMotorControlDevRef"=w193:T7)  [unwired: 7 in, 1 out]
            }
            n122 = call "CTRE_Phoenix_MotorControl_Set.vi"("Output"=0.0, "Control Mode"=w183, "PhoenixMotorControlDevRef"=w184) -> ()  [unwired: 7 in, 2 out]
          }
          frame "Wait" {
            n123 = while {
              tunnel: w217 -> [w219]
              stop <- w218 stop-if-true
              n124 = call "Elapsed Time19"("Time Target (s)"=w219) -> ("Time has Elapsed"=w218:bool)  [unwired: 11 in, 7 out]
            }
          }
          frame "Grab" {
            # "Direction"
            n125 = call <vilib>:"WPI_SolenoidRefNum Registry Get.vi"("refnum name"="Claw") -> ("SolenoidDevRef"=w224:T12)  [unwired: 9 in, 1 out]
            n126 = Equal?(x=w227, y=0.0) -> (x = y?=w225:bool)
            n127 = Select(t=WPI_SolenoidValue."Reverse" ("Value"), s=w225, f=WPI_SolenoidValue."Forward") -> (s? t:f=w222:T3)
            n128 = call-poly <vilib>:"WPI_SolenoidSet.vi"("Value"=w222, "SolenoidDevRef"=w224) -> ()  [unwired: 8 in, 2 out]
          }
        }
      }
    }
    frame "Center" {
      n129 = call "CTRE_Phoenix_MotorControl_RefNumRegistryGet.vi"("refnum name"="Elevator") -> ("PhoenixMotorControlDevRef"=w230:T7)  [unwired: 9 in, 1 out]
      n130 = flat-sequence {
        tunnel: w275 -> [w282]
        tunnel: [w281] -> w274
        tunnel: [w280] -> w273
        tunnel: w272 -> [w280]
        tunnel: w271 -> [w279]
        tunnel: [w279] -> w270
        tunnel: w230 -> [w276]
        tunnel: w274 -> [w288]
        tunnel: w273 -> [w287]
        tunnel: w270 -> [w286]
        tunnel: [w285] -> w261
        tunnel: [w284] -> w259
        tunnel: [w283] -> w257
        tunnel: w261 -> [w309]
        tunnel: [w309] -> w260
        tunnel: w259 -> [w305]
        tunnel: [w305] -> w258
        tunnel: w257 -> [w304]
        tunnel: [w304] -> w256
        tunnel: w260 -> [w313]
        tunnel: [w313] -> w265
        tunnel: w258 -> [w312]
        tunnel: [w312] -> w264
        tunnel: w256 -> [w311]
        tunnel: [w311] -> w263
        tunnel: [w310] -> w262
        tunnel: [w332] -> w269
        tunnel: w265 -> [w332]
        tunnel: w264 -> [w331]
        tunnel: [w331] -> w268
        tunnel: [w330] -> w267
        tunnel: w263 -> [w330]
        tunnel: w262 -> [w327]
        tunnel: [w323] -> w266
        tunnel: w269 -> [w340]
        tunnel: w268 -> [w339]
        tunnel: w267 -> [w338]
        tunnel: [w337] -> w247
        tunnel: [w336] -> w245
        tunnel: [w335] -> w243
        tunnel: w266 -> [w334]
        tunnel: [w334] -> w241
        tunnel: w247 -> [w354]
        tunnel: [w354] -> w246
        tunnel: w245 -> [w355]
        tunnel: [w355] -> w244
        tunnel: w243 -> [w358]
        tunnel: [w358] -> w242
        tunnel: w241 -> [w359]
        tunnel: [w359] -> w240
        tunnel: w246 -> [w366]
        tunnel: w244 -> [w365]
        tunnel: w242 -> [w364]
        tunnel: [w363] -> w255
        tunnel: [w362] -> w253
        tunnel: [w361] -> w251
        tunnel: w240 -> [w360]
        tunnel: [w360] -> w249
        tunnel: w255 -> [w387]
        tunnel: [w387] -> w254
        tunnel: w253 -> [w386]
        tunnel: [w386] -> w252
        tunnel: w251 -> [w394]
        tunnel: [w394] -> w250
        tunnel: w249 -> [w393]
        tunnel: [w393] -> w248
        tunnel: w254 -> [w401]
        tunnel: w252 -> [w400]
        tunnel: w250 -> [w399]
        tunnel: [w398] -> w239
        tunnel: [w397] -> w237
        tunnel: [w396] -> w235
        tunnel: w248 -> [w395]
        tunnel: w239 -> [w416]
        tunnel: [w416] -> w238
        tunnel: w237 -> [w417]
        tunnel: [w417] -> w236
        tunnel: w235 -> [w415]
        tunnel: [w415] -> w234
        tunnel: w238 -> [w424]
        tunnel: w236 -> [w423]
        tunnel: w234 -> [w422]
        tunnel: [w421] -> w233
        tunnel: [w420] -> w232
        tunnel: w233 -> [w444]
        tunnel: w232 -> [w443]
        tunnel: [w445] -> w229
        tunnel: w229 -> [w472]
        tunnel: [w471] -> w228
        tunnel: w228 -> [w480]
        frame #0 {
          w278 = T16 0 items=["PercentOutput"=0, "Position"=1, "Velocity"=2, "Current"=3, "Follower"=5, "MotionProfile"=6, "MotionMagic"=7, "MotionMagicArc"=8, "MotionProfileArc"=10, "Disabled"=15] ("Control Mode")
          n131 = call "Z900_navX_Set_ZeroYaw.vi"("navX Device"=w282) -> ("navX Device"=w281:T14)  [unwired: 9 in, 1 out]
          n132 = call "CTRE_Phoenix_MotorControl_Set.vi"("Output"=-0.1, "Control Mode"=w278, "PhoenixMotorControlDevRef"=w276) -> ()  [unwired: 7 in, 2 out]
        }
        frame #1 {
          n133 = while {
            tunnel: w288 -> [w300]
            tunnel: w287 -> [w299]
            tunnel: w286 -> [w298]
            tunnel: [w300] -> w285
            tunnel: [w299] -> w284
            tunnel: [w298] -> w283
            stop <- w294 stop-if-true
            n134 = call "GoDistance.vi"("Forward PID"="forward PID", "Angle PID"="angle PID", "x"=2.0, "PhoenixMotorControlDevRef"=w298, "PhoenixMotorControlDevRef 2"=w299, "navX Device"=w300) -> ("Error 2"=w290:dbl, "Error 1"=w295:dbl)  [unwired: 4 in]
            n135 = Less?(x=w295, y=60.0) -> (x < y?=w292:bool)
            n136 = Less?(x=w290, y=3.0) -> (x < y?=w289:bool)
            n137 = And(x=w292, y=w289) -> (x .and. y?=w294:bool)
          }
        }
        frame #2 {
          w306 = 0.0 ("Output")
          w307 = T16 0 items=["PercentOutput"=0, "Position"=1, "Velocity"=2, "Current"=3, "Follower"=5, "MotionProfile"=6, "MotionMagic"=7, "MotionMagicArc"=8, "MotionProfileArc"=10, "Disabled"=15] ("Control Mode")
          w308 = T16 0 items=["PercentOutput"=0, "Position"=1, "Velocity"=2, "Current"=3, "Follower"=5, "MotionProfile"=6, "MotionMagic"=7, "MotionMagicArc"=8, "MotionProfileArc"=10, "Disabled"=15] ("Control Mode")
          n138 = call "CTRE_Phoenix_MotorControl_SetSelectedSensorPosition.vi"("New Sensor Position"=0, "PhoenixMotorControlDevRef"=w304) -> ()  [unwired: 8 in, 2 out]
          n139 = call "CTRE_Phoenix_MotorControl_SetSelectedSensorPosition.vi"("New Sensor Position"=0, "PhoenixMotorControlDevRef"=w305) -> ()  [unwired: 8 in, 2 out]
          n140 = call "CTRE_Phoenix_MotorControl_Set.vi"("Output"=w306, "Control Mode"=w308, "PhoenixMotorControlDevRef"=w304) -> ()  [unwired: 7 in, 2 out]
          n141 = call "CTRE_Phoenix_MotorControl_Set.vi"("Output"=w306, "Control Mode"=w307, "PhoenixMotorControlDevRef"=w305) -> ()  [unwired: 7 in, 2 out]
        }
        frame #3 {
          n142 = while {
            tunnel: [w318] -> w310
            stop <- w314 stop-if-true
            n143 = call <vilib>:"WPI_DriverStationGame Specific Data.vi"() -> ("Game Specific Data"=w318:string)  [unwired: 11 in]
            n144 = call "Elapsed Time2"("Time Target (s)"=2.0) -> ("Time has Elapsed"=w315:bool)  [unwired: 11 in, 7 out]
            n145 = String Length(string=w318) -> (length=w320:i32)
            n146 = Greater?(x=w320, y=0) -> (0:w316:bool)
            n147 = Or(x=w316, y=w315) -> (x .or. y?=w314:bool)
          }
        }
        frame #4 {
          n148 = String Subset(string=w327, offset (0)=0, length (rest)=1 ("length (rest)")) -> (substring=w326:string)
          n149 = Wait (ms)(milliseconds to wait=u32 500) -> ()  [unwired: 1 out]
          n150 = Equal?(x=w326, y="L") -> (x = y?=w324:bool)
          n151 = Select(t=-1.0, s=w324, f=1.0) -> (s? t:f=w323:dbl)
        }
        frame #5 {
          n152 = while {
            tunnel: w340 -> [w353]
            tunnel: w339 -> [w350]
            tunnel: w338 -> [w351]
            tunnel: [w349] -> w337
            tunnel: [w348] -> w336
            tunnel: [w347] -> w335
            tunnel: w334 -> [w342]
            stop <- w344 stop-if-true
            n153 = local read "angle PID"() -> (w352:T2)
            n154 = Multiply(x=90.0 ("setpoint"), y=w342) -> (x*y=w341:dbl)
            n155 = call "RotateToAngle.vi"("setpoint"=w341, "PID gains"=w352, "PhoenixMotorControlDevRef 2"=w350, "PhoenixMotorControlDevRef"=w351, "navX Device"=w353) -> ("abs(x)"=w346:dbl, "PhoenixMotorControlDevRef 3"=w349:T7, "PhoenixMotorControlDevRef 4"=w348:T7, "navX Device 2"=w347:T14)  [unwired: 3 in]
            n156 = Less?(x=w346, y=5.0) -> (x < y?=w344:bool)
          }
        }
        frame #6 {
          n157 = call "Z900_navX_Set_ZeroYaw.vi"("navX Device"=w358) -> ()  [unwired: 9 in, 2 out]
          n158 = call "CTRE_Phoenix_MotorControl_SetSelectedSensorPosition.vi"("New Sensor Position"=0, "PhoenixMotorControlDevRef"=w354) -> ()  [unwired: 8 in, 2 out]
          n159 = call "CTRE_Phoenix_MotorControl_SetSelectedSensorPosition.vi"("New Sensor Position"=0, "PhoenixMotorControlDevRef"=w355) -> ()  [unwired: 8 in, 2 out]
        }
        frame #7 {
          n160 = while {
            tunnel: w366 -> [w374]
            tunnel: w365 -> [w375]
            tunnel: w364 -> [w373]
            tunnel: [w375] -> w363
            tunnel: [w374] -> w362
            tunnel: [w373] -> w361
            tunnel: w360 -> [w372]
            stop <- w379 stop-if-true
            n161 = local read "forward PID"() -> (w383:T2)
            n162 = local read "angle PID"() -> (w384:T2)
            n163 = Negate(x=w372) -> (-x=w371:dbl)
            n164 = Multiply(x=0.5, y=w371) -> (x*y=w368:dbl)
            n165 = Add(x=4.7, y=w368) -> (x+y=w367:dbl)
            n166 = call "GoDistance.vi"("Forward PID"=w383, "Angle PID"=w384, "x"=w367, "PhoenixMotorControlDevRef"=w375, "PhoenixMotorControlDevRef 2"=w374, "navX Device"=w373) -> ("Error 2"=w376:dbl, "Error 1"=w378:dbl)  [unwired: 4 in]
            n167 = Less?(x=w376, y=4.0) -> (x < y?=w380:bool)
            n168 = Less?(x=w378, y=60.0) -> (x < y?=w381:bool)
            n169 = And(x=w381, y=w380) -> (x .and. y?=w379:bool)
          }
        }
        frame #8 {
          w390 = 0.0 ("Output")
          w391 = T16 0 items=["PercentOutput"=0, "Position"=1, "Velocity"=2, "Current"=3, "Follower"=5, "MotionProfile"=6, "MotionMagic"=7, "MotionMagicArc"=8, "MotionProfileArc"=10, "Disabled"=15] ("Control Mode")
          w392 = T16 0 items=["PercentOutput"=0, "Position"=1, "Velocity"=2, "Current"=3, "Follower"=5, "MotionProfile"=6, "MotionMagic"=7, "MotionMagicArc"=8, "MotionProfileArc"=10, "Disabled"=15] ("Control Mode")
          n170 = Wait (ms)(milliseconds to wait=u32 500) -> ()  [unwired: 1 out]
          n171 = call "CTRE_Phoenix_MotorControl_SetSelectedSensorPosition.vi"("New Sensor Position"=0, "PhoenixMotorControlDevRef"=w387) -> ()  [unwired: 8 in, 2 out]
          n172 = call "CTRE_Phoenix_MotorControl_SetSelectedSensorPosition.vi"("New Sensor Position"=0, "PhoenixMotorControlDevRef"=w386) -> ()  [unwired: 8 in, 2 out]
          n173 = call "CTRE_Phoenix_MotorControl_Set.vi"("Output"=w390, "Control Mode"=w392, "PhoenixMotorControlDevRef"=w387) -> ()  [unwired: 7 in, 2 out]
          n174 = call "CTRE_Phoenix_MotorControl_Set.vi"("Output"=w390, "Control Mode"=w391, "PhoenixMotorControlDevRef"=w386) -> ()  [unwired: 7 in, 2 out]
        }
        frame #9 {
          n175 = while {
            tunnel: w401 -> [w414]
            tunnel: w400 -> [w413]
            tunnel: w399 -> [w412]
            tunnel: [w407] -> w398
            tunnel: [w406] -> w397
            tunnel: [w405] -> w396
            tunnel: w395 -> [w402]
            stop <- w408 stop-if-true
            n176 = local read "angle PID"() -> (w411:T2)
            n177 = Multiply(x=-90.0 ("setpoint"), y=w402) -> (x*y=w403:dbl)
            n178 = call "RotateToAngle.vi"("setpoint"=w403, "PID gains"=w411, "PhoenixMotorControlDevRef 2"=w413, "PhoenixMotorControlDevRef"=w414, "navX Device"=w412) -> ("abs(x)"=w409:dbl, "PhoenixMotorControlDevRef 3"=w406:T7, "PhoenixMotorControlDevRef 4"=w407:T7, "navX Device 2"=w405:T14)  [unwired: 3 in]
            n179 = Less?(x=w409, y=5.0) -> (x < y?=w408:bool)
          }
        }
        frame #10 {
          n180 = call "Z900_navX_Set_ZeroYaw.vi"("navX Device"=w415) -> ()  [unwired: 9 in, 2 out]
          n181 = call "CTRE_Phoenix_MotorControl_SetSelectedSensorPosition.vi"("New Sensor Position"=0, "PhoenixMotorControlDevRef"=w416) -> ()  [unwired: 8 in, 2 out]
          n182 = call "CTRE_Phoenix_MotorControl_SetSelectedSensorPosition.vi"("New Sensor Position"=0, "PhoenixMotorControlDevRef"=w417) -> ()  [unwired: 8 in, 2 out]
        }
        frame #11 {
          n183 = while {
            tunnel: w424 -> [w426]
            tunnel: w423 -> [w425]
            tunnel: w422 -> [w440]
            tunnel: [w426] -> w421
            tunnel: [w425] -> w420
            stop <- w427 stop-if-true
            n184 = call "Elapsed Time4"("Time Target (s)"=3.0) -> ("Time has Elapsed"=w428:bool)  [unwired: 11 in, 7 out]
            n185 = local read "angle PID"() -> (w439:T2)
            n186 = local read "forward PID"() -> (w437:T2)
            n187 = call "GoDistance.vi"("Forward PID"=w437, "Angle PID"=w439, "x"=10.0, "PhoenixMotorControlDevRef"=w426, "PhoenixMotorControlDevRef 2"=w425, "navX Device"=w440) -> ("Error 2"=w431:dbl, "Error 1"=w432:dbl)  [unwired: 4 in]
            n188 = Less?(x=w431, y=4.0) -> (x < y?=w434:bool)
            n189 = Less?(x=w432, y=60.0) -> (x < y?=w435:bool)
            n190 = And(x=w435, y=w434) -> (x .and. y?=w429:bool)
            n191 = Or(x=w429, y=w428) -> (x .or. y?=w427:bool)
          }
        }
        frame #12 {
          w442 = T16 0 items=["PercentOutput"=0, "Position"=1, "Velocity"=2, "Current"=3, "Follower"=5, "MotionProfile"=6, "MotionMagic"=7, "MotionMagicArc"=8, "MotionProfileArc"=10, "Disabled"=15] ("Control Mode")
          w441 = 0.0 ("Output")
          n192 = call "CTRE_Phoenix_MotorControl_Set.vi"("Output"=w441, "Control Mode"=w442, "PhoenixMotorControlDevRef"=w443) -> ()  [unwired: 7 in, 2 out]
          n193 = call "CTRE_Phoenix_MotorControl_Set.vi"("Output"=w441, "Control Mode"=w442, "PhoenixMotorControlDevRef"=w444) -> ()  [unwired: 7 in, 2 out]
        }
        frame #13 {
          n194 = call "CTRE_Phoenix_MotorControl_RefNumRegistryGet.vi"("refnum name"="Elevator") -> ("PhoenixMotorControlDevRef"=w446:T7)  [unwired: 9 in, 1 out]
          n195 = while {
            tunnel: w446 -> [w453]
            tunnel: [w449] -> w445
            stop <- w450 stop-if-true
            w454 = T16 0 items=["PercentOutput"=0, "Position"=1, "Velocity"=2, "Current"=3, "Follower"=5, "MotionProfile"=6, "MotionMagic"=7, "MotionMagicArc"=8, "MotionProfileArc"=10, "Disabled"=15] ("Control Mode")
            n196 = disable-structure shown="Disabled" {
              disable-tunnel: w453 -> [w455 _]
              frame Disabled {
                n197 = call-poly "CTRE_Phoenix_MotorController_Get_Enhanced.vi"("PhoenixMotorControlDevRef"=w455) -> ("Position (Raw Sensor Units)"=w457:i32)  [unwired: 11 in, 3 out]
                n198 = Subtract(x="elevatorPosition", y=w457) -> (x-y=w461:dbl)
                n199 = Absolute Value(x=w461) -> (abs(x)=w460:dbl)
                n200 = call-poly "CTRE_Phoenix_MotorController_Get_Enhanced.vi"("PhoenixMotorControlDevRef"=w455) -> ()  [unwired: 11 in, 4 out]
                n201 = Less?(x=w460, y=10.0) -> ()  [unwired: 1 out]
                n202 = call-poly <vilib>:"PID.vi"("output range"=cluster{"output high":dbl, "output low":dbl} {"output high"=0.7, "output low"=-0.7}, "PID gains"="elevator PID", "process variable"=w457, "setpoint"="elevatorPosition") -> ("output"=w456:dbl)  [unwired: 6 in, 1 out]
                n203 = Negate(x=w456) -> ()  [unwired: 1 out]
              }
              frame Enabled {
              }
            }
            n204 = call "Elapsed Time7"("Time Target (s)"=0.3) -> ("Time has Elapsed"=w450:bool)  [unwired: 11 in, 7 out]
            n205 = call "CTRE_Phoenix_MotorControl_Set.vi"("Output"=0.5, "Control Mode"=w454, "PhoenixMotorControlDevRef"=w453) -> ("PhoenixMotorControlDevRef"=w449:T7)  [unwired: 7 in, 1 out]
            n206 = case shown="True" FALSE {
              frame False {
              }
              frame True {
                w464 = T16 0 items=["PercentOutput"=0, "Position"=1, "Velocity"=2, "Current"=3, "Follower"=5, "MotionProfile"=6, "MotionMagic"=7, "MotionMagicArc"=8, "MotionProfileArc"=10, "Disabled"=15] ("Control Mode")
                w465 = 1.0 ("Output")
                n207 = call "CTRE_Phoenix_MotorControl_RefNumRegistryGet.vi"("refnum name"="IOL") -> ("PhoenixMotorControlDevRef"=w468:T7)  [unwired: 9 in, 1 out]
                n208 = call "CTRE_Phoenix_MotorControl_RefNumRegistryGet.vi"("refnum name"="IOR") -> ("PhoenixMotorControlDevRef"=w467:T7)  [unwired: 9 in, 1 out]
                n209 = call "Elapsed Time"("Time Target (s)"=2.0) -> ()  [unwired: 11 in, 8 out]
                n210 = call "CTRE_Phoenix_MotorControl_Set.vi"("Output"=w465, "Control Mode"=w464, "PhoenixMotorControlDevRef"=w468) -> ()  [unwired: 7 in, 2 out]
                n211 = call "CTRE_Phoenix_MotorControl_Set.vi"("Output"=w465, "Control Mode"=w464, "PhoenixMotorControlDevRef"=w467) -> ()  [unwired: 7 in, 2 out]
              }
            }
          }
        }
        frame #14 {
          n212 = while {
            tunnel: w472 -> [w474]
            tunnel: [w475] -> w471
            stop <- w473 stop-if-true
            w477 = T16 0 items=["PercentOutput"=0, "Position"=1, "Velocity"=2, "Current"=3, "Follower"=5, "MotionProfile"=6, "MotionMagic"=7, "MotionMagicArc"=8, "MotionProfileArc"=10, "Disabled"=15] ("Control Mode")
            n213 = call "CTRE_Phoenix_MotorControl_Set.vi"("Output"=0.0, "Control Mode"=w477, "PhoenixMotorControlDevRef"=w474) -> ("PhoenixMotorControlDevRef"=w475:T7)  [unwired: 7 in, 1 out]
            n214 = call-poly "CTRE_Phoenix_MotorController_Get_Enhanced.vi"("PhoenixMotorControlDevRef"=w474) -> ("Reverse Limit Closed?"=w473:bool)  [unwired: 11 in, 3 out]
          }
        }
        frame #15 {
          w482 = T16 0 items=["PercentOutput"=0, "Position"=1, "Velocity"=2, "Current"=3, "Follower"=5, "MotionProfile"=6, "MotionMagic"=7, "MotionMagicArc"=8, "MotionProfileArc"=10, "Disabled"=15] ("Control Mode")
          n215 = call "CTRE_Phoenix_MotorControl_SetSelectedSensorPosition.vi"("New Sensor Position"=0, "PhoenixMotorControlDevRef"=w480) -> ("PhoenixMotorControlDevRef"=w479:T7)  [unwired: 8 in, 1 out]
          n216 = call "CTRE_Phoenix_MotorControl_Set.vi"("Output"=0.0, "Control Mode"=w482, "PhoenixMotorControlDevRef"=w479) -> ()  [unwired: 7 in, 2 out]
        }
      }
    }
    frame "Center Elbow" {
      n217 = call "Z900_navX_Set_ZeroYaw.vi"("navX Device"=w487) -> ("navX Device"=w486:T14)  [unwired: 9 in, 1 out]
      n218 = flat-sequence {
        tunnel: w486 -> [w533]
        tunnel: w528 -> [w534]
        tunnel: w527 -> [w535]
        tunnel: [w535] -> w485
        tunnel: [w534] -> w484
        tunnel: [w533] -> w483
        tunnel: [w539] -> w518
        tunnel: [w538] -> w516
        tunnel: [w537] -> w514
        tunnel: w485 -> [w540]
        tunnel: w484 -> [w541]
        tunnel: w483 -> [w536]
        tunnel: w518 -> [w562]
        tunnel: [w562] -> w517
        tunnel: w516 -> [w558]
        tunnel: [w558] -> w515
        tunnel: w514 -> [w557]
        tunnel: [w557] -> w513
        tunnel: w517 -> [w566]
        tunnel: [w566] -> w522
        tunnel: w515 -> [w565]
        tunnel: [w565] -> w521
        tunnel: w513 -> [w564]
        tunnel: [w564] -> w520
        tunnel: [w563] -> w519
        tunnel: [w585] -> w526
        tunnel: w522 -> [w585]
        tunnel: w521 -> [w584]
        tunnel: [w584] -> w525
        tunnel: [w583] -> w524
        tunnel: w520 -> [w583]
        tunnel: w519 -> [w580]
        tunnel: [w576] -> w523
        tunnel: w526 -> [w593]
        tunnel: w525 -> [w592]
        tunnel: w524 -> [w591]
        tunnel: [w590] -> w504
        tunnel: [w589] -> w502
        tunnel: [w588] -> w500
        tunnel: w523 -> [w587]
        tunnel: [w587] -> w498
        tunnel: w504 -> [w607]
        tunnel: [w607] -> w503
        tunnel: w502 -> [w608]
        tunnel: [w608] -> w501
        tunnel: w500 -> [w611]
        tunnel: [w611] -> w499
        tunnel: w498 -> [w612]
        tunnel: [w612] -> w497
        tunnel: w503 -> [w619]
        tunnel: w501 -> [w618]
        tunnel: w499 -> [w617]
        tunnel: [w616] -> w512
        tunnel: [w615] -> w510
        tunnel: [w614] -> w508
        tunnel: w497 -> [w613]
        tunnel: [w613] -> w506
        tunnel: w512 -> [w635]
        tunnel: [w635] -> w511
        tunnel: w510 -> [w634]
        tunnel: [w634] -> w509
        tunnel: w508 -> [w642]
        tunnel: [w642] -> w507
        tunnel: w506 -> [w641]
        tunnel: [w641] -> w505
        tunnel: w511 -> [w649]
        tunnel: w509 -> [w648]
        tunnel: w507 -> [w647]
        tunnel: [w646] -> w496
        tunnel: [w645] -> w494
        tunnel: [w644] -> w492
        tunnel: w505 -> [w643]
        tunnel: w496 -> [w664]
        tunnel: [w664] -> w495
        tunnel: w494 -> [w665]
        tunnel: [w665] -> w493
        tunnel: w492 -> [w663]
        tunnel: [w663] -> w491
        tunnel: w495 -> [w672]
        tunnel: w493 -> [w671]
        tunnel: w491 -> [w670]
        tunnel: [w669] -> w490
        tunnel: [w668] -> w489
        tunnel: w490 -> [w692]
        tunnel: w489 -> [w691]
        tunnel: [w693] -> w488
        tunnel: w488 -> [w720]
        frame #0 {
          n219 = call <vilib>:"WPI_SolenoidRefNum Registry Get.vi"("refnum name"="Elbow") -> ("SolenoidDevRef"=w531:T12)  [unwired: 9 in, 1 out]
          n220 = Wait (ms)(milliseconds to wait=u32 250) -> ()  [unwired: 1 out]
          n221 = call-poly <vilib>:"WPI_SolenoidSet.vi"("Value"=WPI_SolenoidValue."Reverse", "SolenoidDevRef"=w531) -> ()  [unwired: 8 in, 2 out]
        }
        frame #1 {
          n222 = while {
            tunnel: w536 -> [w554]
            tunnel: w541 -> [w553]
            tunnel: w540 -> [w552]
            tunnel: [w554] -> w539
            tunnel: [w553] -> w538
            tunnel: [w552] -> w537
            stop <- w549 stop-if-true
            n223 = local read "angle PID"() -> (w542:T2)
            n224 = local read "forward PID"() -> (w543:T2)
            n225 = call "GoDistance.vi"("Forward PID"=w543, "Angle PID"=w542, "x"=2.0, "PhoenixMotorControlDevRef"=w552, "PhoenixMotorControlDevRef 2"=w553, "navX Device"=w554) -> ("Error 2"=w545:dbl, "Error 1"=w550:dbl)  [unwired: 4 in]
            n226 = Less?(x=w550, y=60.0) -> (x < y?=w547:bool)
            n227 = Less?(x=w545, y=3.0) -> (x < y?=w544:bool)
            n228 = And(x=w547, y=w544) -> (x .and. y?=w549:bool)
          }
        }
        frame #2 {
          w559 = 0.0 ("Output")
          w560 = T16 0 items=["PercentOutput"=0, "Position"=1, "Velocity"=2, "Current"=3, "Follower"=5, "MotionProfile"=6, "MotionMagic"=7, "MotionMagicArc"=8, "MotionProfileArc"=10, "Disabled"=15] ("Control Mode")
          w561 = T16 0 items=["PercentOutput"=0, "Position"=1, "Velocity"=2, "Current"=3, "Follower"=5, "MotionProfile"=6, "MotionMagic"=7, "MotionMagicArc"=8, "MotionProfileArc"=10, "Disabled"=15] ("Control Mode")
          n229 = call "CTRE_Phoenix_MotorControl_SetSelectedSensorPosition.vi"("New Sensor Position"=0, "PhoenixMotorControlDevRef"=w557) -> ()  [unwired: 8 in, 2 out]
          n230 = call "CTRE_Phoenix_MotorControl_SetSelectedSensorPosition.vi"("New Sensor Position"=0, "PhoenixMotorControlDevRef"=w558) -> ()  [unwired: 8 in, 2 out]
          n231 = call "CTRE_Phoenix_MotorControl_Set.vi"("Output"=w559, "Control Mode"=w561, "PhoenixMotorControlDevRef"=w557) -> ()  [unwired: 7 in, 2 out]
          n232 = call "CTRE_Phoenix_MotorControl_Set.vi"("Output"=w559, "Control Mode"=w560, "PhoenixMotorControlDevRef"=w558) -> ()  [unwired: 7 in, 2 out]
        }
        frame #3 {
          n233 = while {
            tunnel: [w571] -> w563
            stop <- w567 stop-if-true
            n234 = call <vilib>:"WPI_DriverStationGame Specific Data.vi"() -> ("Game Specific Data"=w571:string)  [unwired: 11 in]
            n235 = call "Elapsed Time13"("Time Target (s)"=2.0) -> ("Time has Elapsed"=w568:bool)  [unwired: 11 in, 7 out]
            n236 = String Length(string=w571) -> (length=w573:i32)
            n237 = Greater?(x=w573, y=0) -> (0:w569:bool)
            n238 = Or(x=w569, y=w568) -> (x .or. y?=w567:bool)
          }
        }
        frame #4 {
          n239 = String Subset(string=w580, offset (0)=0, length (rest)=1 ("length (rest)")) -> (substring=w579:string)
          n240 = Wait (ms)(milliseconds to wait=u32 500) -> ()  [unwired: 1 out]
          n241 = Equal?(x=w579, y="L") -> (x = y?=w577:bool)
          n242 = Select(t=-1.0, s=w577, f=1.0) -> (s? t:f=w576:dbl)
        }
        frame #5 {
          n243 = while {
            tunnel: w593 -> [w606]
            tunnel: w592 -> [w604]
            tunnel: w591 -> [w605]
            tunnel: [w603] -> w590
            tunnel: [w602] -> w589
            tunnel: [w601] -> w588
            tunnel: w587 -> [w596]
            stop <- w598 stop-if-true
            n244 = local read "angle PID"() -> (w594:T2)
            n245 = Multiply(x=90.0 ("setpoint"), y=w596) -> (x*y=w595:dbl)
            n246 = call "RotateToAngle.vi"("setpoint"=w595, "PID gains"=w594, "PhoenixMotorControlDevRef 2"=w604, "PhoenixMotorControlDevRef"=w605, "navX Device"=w606) -> ("abs(x)"=w600:dbl, "PhoenixMotorControlDevRef 3"=w603:T7, "PhoenixMotorControlDevRef 4"=w602:T7, "navX Device 2"=w601:T14)  [unwired: 3 in]
            n247 = Less?(x=w600, y=5.0) -> (x < y?=w598:bool)
          }
        }
        frame #6 {
          n248 = call "Z900_navX_Set_ZeroYaw.vi"("navX Device"=w611) -> ()  [unwired: 9 in, 2 out]
          n249 = call "CTRE_Phoenix_MotorControl_SetSelectedSensorPosition.vi"("New Sensor Position"=0, "PhoenixMotorControlDevRef"=w607) -> ()  [unwired: 8 in, 2 out]
          n250 = call "CTRE_Phoenix_MotorControl_SetSelectedSensorPosition.vi"("New Sensor Position"=0, "PhoenixMotorControlDevRef"=w608) -> ()  [unwired: 8 in, 2 out]
        }
        frame #7 {
          n251 = while {
            tunnel: w619 -> [w623]
            tunnel: w618 -> [w624]
            tunnel: w617 -> [w622]
            tunnel: [w624] -> w616
            tunnel: [w623] -> w615
            tunnel: [w622] -> w614
            stop <- w628 stop-if-true
            n252 = local read "forward PID"() -> (w621:T2)
            n253 = local read "angle PID"() -> (w620:T2)
            n254 = call "GoDistance.vi"("Forward PID"=w621, "Angle PID"=w620, "x"=4.0, "PhoenixMotorControlDevRef"=w624, "PhoenixMotorControlDevRef 2"=w623, "navX Device"=w622) -> ("Error 2"=w625:dbl, "Error 1"=w627:dbl)  [unwired: 4 in]
            n255 = Less?(x=w625, y=4.0) -> (x < y?=w629:bool)
            n256 = Less?(x=w627, y=60.0) -> (x < y?=w630:bool)
            n257 = And(x=w630, y=w629) -> (x .and. y?=w628:bool)
          }
        }
        frame #8 {
          w638 = 0.0 ("Output")
          w639 = T16 0 items=["PercentOutput"=0, "Position"=1, "Velocity"=2, "Current"=3, "Follower"=5, "MotionProfile"=6, "MotionMagic"=7, "MotionMagicArc"=8, "MotionProfileArc"=10, "Disabled"=15] ("Control Mode")
          w640 = T16 0 items=["PercentOutput"=0, "Position"=1, "Velocity"=2, "Current"=3, "Follower"=5, "MotionProfile"=6, "MotionMagic"=7, "MotionMagicArc"=8, "MotionProfileArc"=10, "Disabled"=15] ("Control Mode")
          n258 = Wait (ms)(milliseconds to wait=u32 500) -> ()  [unwired: 1 out]
          n259 = call "CTRE_Phoenix_MotorControl_SetSelectedSensorPosition.vi"("New Sensor Position"=0, "PhoenixMotorControlDevRef"=w635) -> ()  [unwired: 8 in, 2 out]
          n260 = call "CTRE_Phoenix_MotorControl_SetSelectedSensorPosition.vi"("New Sensor Position"=0, "PhoenixMotorControlDevRef"=w634) -> ()  [unwired: 8 in, 2 out]
          n261 = call "CTRE_Phoenix_MotorControl_Set.vi"("Output"=w638, "Control Mode"=w640, "PhoenixMotorControlDevRef"=w635) -> ()  [unwired: 7 in, 2 out]
          n262 = call "CTRE_Phoenix_MotorControl_Set.vi"("Output"=w638, "Control Mode"=w639, "PhoenixMotorControlDevRef"=w634) -> ()  [unwired: 7 in, 2 out]
        }
        frame #9 {
          n263 = while {
            tunnel: w649 -> [w662]
            tunnel: w648 -> [w661]
            tunnel: w647 -> [w660]
            tunnel: [w656] -> w646
            tunnel: [w655] -> w645
            tunnel: [w654] -> w644
            tunnel: w643 -> [w651]
            stop <- w657 stop-if-true
            n264 = local read "angle PID"() -> (w650:T2)
            n265 = Multiply(x=-90.0 ("setpoint"), y=w651) -> (x*y=w652:dbl)
            n266 = call "RotateToAngle.vi"("setpoint"=w652, "PID gains"=w650, "PhoenixMotorControlDevRef 2"=w661, "PhoenixMotorControlDevRef"=w662, "navX Device"=w660) -> ("abs(x)"=w658:dbl, "PhoenixMotorControlDevRef 3"=w655:T7, "PhoenixMotorControlDevRef 4"=w656:T7, "navX Device 2"=w654:T14)  [unwired: 3 in]
            n267 = Less?(x=w658, y=5.0) -> (x < y?=w657:bool)
          }
        }
        frame #10 {
          n268 = call "Z900_navX_Set_ZeroYaw.vi"("navX Device"=w663) -> ()  [unwired: 9 in, 2 out]
          n269 = call "CTRE_Phoenix_MotorControl_SetSelectedSensorPosition.vi"("New Sensor Position"=0, "PhoenixMotorControlDevRef"=w664) -> ()  [unwired: 8 in, 2 out]
          n270 = call "CTRE_Phoenix_MotorControl_SetSelectedSensorPosition.vi"("New Sensor Position"=0, "PhoenixMotorControlDevRef"=w665) -> ()  [unwired: 8 in, 2 out]
        }
        frame #11 {
          n271 = while {
            tunnel: w672 -> [w676]
            tunnel: w671 -> [w675]
            tunnel: w670 -> [w688]
            tunnel: [w676] -> w669
            tunnel: [w675] -> w668
            stop <- w677 stop-if-true
            n272 = call "Elapsed Time10"("Time Target (s)"=3.0) -> ("Time has Elapsed"=w678:bool)  [unwired: 11 in, 7 out]
            n273 = local read "angle PID"() -> (w674:T2)
            n274 = local read "forward PID"() -> (w673:T2)
            n275 = call "GoDistance.vi"("Forward PID"=w673, "Angle PID"=w674, "x"=10.0, "PhoenixMotorControlDevRef"=w676, "PhoenixMotorControlDevRef 2"=w675, "navX Device"=w688) -> ("Error 2"=w681:dbl, "Error 1"=w682:dbl)  [unwired: 4 in]
            n276 = Less?(x=w681, y=4.0) -> (x < y?=w684:bool)
            n277 = Less?(x=w682, y=60.0) -> (x < y?=w685:bool)
            n278 = And(x=w685, y=w684) -> (x .and. y?=w679:bool)
            n279 = Or(x=w679, y=w678) -> (x .or. y?=w677:bool)
          }
        }
        frame #12 {
          w690 = T16 0 items=["PercentOutput"=0, "Position"=1, "Velocity"=2, "Current"=3, "Follower"=5, "MotionProfile"=6, "MotionMagic"=7, "MotionMagicArc"=8, "MotionProfileArc"=10, "Disabled"=15] ("Control Mode")
          w689 = 0.0 ("Output")
          n280 = call "CTRE_Phoenix_MotorControl_Set.vi"("Output"=w689, "Control Mode"=w690, "PhoenixMotorControlDevRef"=w691) -> ()  [unwired: 7 in, 2 out]
          n281 = call "CTRE_Phoenix_MotorControl_Set.vi"("Output"=w689, "Control Mode"=w690, "PhoenixMotorControlDevRef"=w692) -> ()  [unwired: 7 in, 2 out]
        }
        frame #13 {
          n282 = call "CTRE_Phoenix_MotorControl_RefNumRegistryGet.vi"("refnum name"="Elevator") -> ("PhoenixMotorControlDevRef"=w694:T7)  [unwired: 9 in, 1 out]
          n283 = while {
            tunnel: w694 -> [w702]
            tunnel: [w702] -> w693
            stop <- w696 stop-if-true
            w701 = T16 0 items=["PercentOutput"=0, "Position"=1, "Velocity"=2, "Current"=3, "Follower"=5, "MotionProfile"=6, "MotionMagic"=7, "MotionMagicArc"=8, "MotionProfileArc"=10, "Disabled"=15] ("Control Mode")
            n284 = local read "elevatorPosition"() -> (w703:dbl)
            n285 = local read "angle PID"() -> (w704:T2)
            n286 = call-poly "CTRE_Phoenix_MotorController_Get_Enhanced.vi"("PhoenixMotorControlDevRef"=w702) -> ("Position (Raw Sensor Units)"=w706:i32)  [unwired: 11 in, 3 out]
            n287 = Subtract(x=w703, y=w706) -> (x-y=w709:dbl)
            n288 = Absolute Value(x=w709) -> (abs(x)=w708:dbl)
            n289 = call-poly "CTRE_Phoenix_MotorController_Get_Enhanced.vi"("PhoenixMotorControlDevRef"=w702) -> ("Reverse Limit Closed?"=w697:bool)  [unwired: 11 in, 3 out]
            n290 = Less?(x=w708, y=10.0) -> (x < y?=w698:bool)
            n291 = call-poly <vilib>:"PID.vi"("output range"=cluster{"output high":dbl, "output low":dbl} {"output high"=0.7, "output low"=-0.7}, "PID gains"=w704, "process variable"=w706, "setpoint"=w703) -> ("output"=w705:dbl)  [unwired: 6 in, 1 out]
            n292 = Negate(x=w705) -> (-x=w700:dbl)
            n293 = call "CTRE_Phoenix_MotorControl_Set.vi"("Output"=w700, "Control Mode"=w701, "PhoenixMotorControlDevRef"=w702) -> ()  [unwired: 7 in, 2 out]
            n294 = Or(x=w698, y=w697) -> (x .or. y?=w699:bool)
            n295 = case shown="True" w699 {
              tunnel: [FALSE ("Time has Elapsed") w712] -> w696
              frame False {
              }
              frame True {
                w713 = T16 0 items=["PercentOutput"=0, "Position"=1, "Velocity"=2, "Current"=3, "Follower"=5, "MotionProfile"=6, "MotionMagic"=7, "MotionMagicArc"=8, "MotionProfileArc"=10, "Disabled"=15] ("Control Mode")
                w714 = 1.0 ("Output")
                n296 = call "CTRE_Phoenix_MotorControl_RefNumRegistryGet.vi"("refnum name"="IOL") -> ("PhoenixMotorControlDevRef"=w717:T7)  [unwired: 9 in, 1 out]
                n297 = call "CTRE_Phoenix_MotorControl_RefNumRegistryGet.vi"("refnum name"="IOR") -> ("PhoenixMotorControlDevRef"=w716:T7)  [unwired: 9 in, 1 out]
                n298 = call "Elapsed Time11"("Time Target (s)"=2.0) -> ("Time has Elapsed"=w712:bool)  [unwired: 11 in, 7 out]
                n299 = call "CTRE_Phoenix_MotorControl_Set.vi"("Output"=w714, "Control Mode"=w713, "PhoenixMotorControlDevRef"=w717) -> ()  [unwired: 7 in, 2 out]
                n300 = call "CTRE_Phoenix_MotorControl_Set.vi"("Output"=w714, "Control Mode"=w713, "PhoenixMotorControlDevRef"=w716) -> ()  [unwired: 7 in, 2 out]
              }
            }
          }
        }
        frame #14 {
          w724 = T16 0 items=["PercentOutput"=0, "Position"=1, "Velocity"=2, "Current"=3, "Follower"=5, "MotionProfile"=6, "MotionMagic"=7, "MotionMagicArc"=8, "MotionProfileArc"=10, "Disabled"=15] ("Control Mode")
          n301 = call "CTRE_Phoenix_MotorControl_SetSelectedSensorPosition.vi"("New Sensor Position"=0, "PhoenixMotorControlDevRef"=w720) -> ("PhoenixMotorControlDevRef"=w722:T7)  [unwired: 8 in, 1 out]
          n302 = call "CTRE_Phoenix_MotorControl_Set.vi"("Output"=0.0, "Control Mode"=w724, "PhoenixMotorControlDevRef"=w722) -> ()  [unwired: 7 in, 2 out]
        }
      }
    }
    frame "Center Ram" {
      n303 = call "CTRE_Phoenix_MotorControl_RefNumRegistryGet.vi"("refnum name"="Elevator") -> ("PhoenixMotorControlDevRef"=w732:T7)  [unwired: 9 in, 1 out]
      n304 = flat-sequence {
        tunnel: w735 -> [w780]
        tunnel: [w779] -> w773
        tunnel: [w778] -> w772
        tunnel: w734 -> [w778]
        tunnel: w733 -> [w777]
        tunnel: [w777] -> w771
        tunnel: w732 -> [w774]
        tunnel: w773 -> [w786]
        tunnel: w772 -> [w785]
        tunnel: w771 -> [w784]
        tunnel: [w783] -> w770
        tunnel: [w782] -> w769
        tunnel: [w781] -> w768
        tunnel: w770 -> [w807]
        tunnel: [w807] -> w767
        tunnel: w769 -> [w803]
        tunnel: [w803] -> w766
        tunnel: w768 -> [w802]
        tunnel: [w802] -> w765
        tunnel: w767 -> [w811]
        tunnel: [w811] -> w764
        tunnel: w766 -> [w810]
        tunnel: [w810] -> w763
        tunnel: w765 -> [w809]
        tunnel: [w809] -> w762
        tunnel: [w808] -> w761
        tunnel: [w830] -> w760
        tunnel: w764 -> [w830]
        tunnel: w763 -> [w829]
        tunnel: [w829] -> w759
        tunnel: [w828] -> w758
        tunnel: w762 -> [w828]
        tunnel: w761 -> [w825]
        tunnel: [w821] -> w757
        tunnel: w760 -> [w838]
        tunnel: w759 -> [w837]
        tunnel: w758 -> [w836]
        tunnel: [w835] -> w756
        tunnel: [w834] -> w755
        tunnel: [w833] -> w754
        tunnel: w757 -> [w832]
        tunnel: [w832] -> w753
        tunnel: w756 -> [w852]
        tunnel: [w852] -> w752
        tunnel: w755 -> [w853]
        tunnel: [w853] -> w751
        tunnel: w754 -> [w856]
        tunnel: [w856] -> w750
        tunnel: w753 -> [w857]
        tunnel: [w857] -> w749
        tunnel: w752 -> [w864]
        tunnel: w751 -> [w863]
        tunnel: w750 -> [w862]
        tunnel: [w861] -> w748
        tunnel: [w860] -> w747
        tunnel: [w859] -> w746
        tunnel: w749 -> [w858]
        tunnel: [w858] -> w745
        tunnel: w748 -> [w880]
        tunnel: [w880] -> w744
        tunnel: w747 -> [w879]
        tunnel: [w879] -> w743
        tunnel: w746 -> [w887]
        tunnel: [w887] -> w742
        tunnel: w745 -> [w886]
        tunnel: [w886] -> w741
        tunnel: w744 -> [w894]
        tunnel: w743 -> [w893]
        tunnel: w742 -> [w892]
        tunnel: [w891] -> w740
        tunnel: [w890] -> w739
        tunnel: [w889] -> w738
        tunnel: w741 -> [w888]
        tunnel: [w913] -> w737
        tunnel: [w912] -> w736
        tunnel: w738 -> [w909]
        tunnel: w739 -> [w912]
        tunnel: w740 -> [w913]
        tunnel: [w908] -> w729
        tunnel: w737 -> [w920]
        tunnel: w736 -> [w919]
        tunnel: [w916] -> w730
        tunnel: w729 -> [w916]
        tunnel: [w915] -> w728
        tunnel: [w914] -> w727
        tunnel: w730 -> [w924]
        tunnel: w728 -> [w923]
        tunnel: w727 -> [w922]
        tunnel: [w921] -> w726
        tunnel: w726 -> [w951]
        tunnel: [w951] -> w725
        tunnel: w725 -> [w952]
        frame #0 {
          w776 = T16 0 items=["PercentOutput"=0, "Position"=1, "Velocity"=2, "Current"=3, "Follower"=5, "MotionProfile"=6, "MotionMagic"=7, "MotionMagicArc"=8, "MotionProfileArc"=10, "Disabled"=15] ("Control Mode")
          n305 = call "Z900_navX_Set_ZeroYaw.vi"("navX Device"=w780) -> ("navX Device"=w779:T14)  [unwired: 9 in, 1 out]
          n306 = call "CTRE_Phoenix_MotorControl_Set.vi"("Output"=-0.1, "Control Mode"=w776, "PhoenixMotorControlDevRef"=w774) -> ()  [unwired: 7 in, 2 out]
        }
        frame #1 {
          n307 = while {
            tunnel: w786 -> [w799]
            tunnel: w785 -> [w798]
            tunnel: w784 -> [w797]
            tunnel: [w799] -> w783
            tunnel: [w798] -> w782
            tunnel: [w797] -> w781
            stop <- w794 stop-if-true
            n308 = local read "angle PID"() -> (w788:T2)
            n309 = local read "forward PID"() -> (w787:T2)
            n310 = call "GoDistance.vi"("Forward PID"=w787, "Angle PID"=w788, "x"=2.0, "PhoenixMotorControlDevRef"=w797, "PhoenixMotorControlDevRef 2"=w798, "navX Device"=w799) -> ("Error 2"=w790:dbl, "Error 1"=w795:dbl)  [unwired: 4 in]
            n311 = Less?(x=w795, y=60.0) -> (x < y?=w792:bool)
            n312 = Less?(x=w790, y=3.0) -> (x < y?=w789:bool)
            n313 = And(x=w792, y=w789) -> (x .and. y?=w794:bool)
          }
        }
        frame #2 {
          w804 = 0.0 ("Output")
          w805 = T16 0 items=["PercentOutput"=0, "Position"=1, "Velocity"=2, "Current"=3, "Follower"=5, "MotionProfile"=6, "MotionMagic"=7, "MotionMagicArc"=8, "MotionProfileArc"=10, "Disabled"=15] ("Control Mode")
          w806 = T16 0 items=["PercentOutput"=0, "Position"=1, "Velocity"=2, "Current"=3, "Follower"=5, "MotionProfile"=6, "MotionMagic"=7, "MotionMagicArc"=8, "MotionProfileArc"=10, "Disabled"=15] ("Control Mode")
          n314 = call "CTRE_Phoenix_MotorControl_SetSelectedSensorPosition.vi"("New Sensor Position"=0, "PhoenixMotorControlDevRef"=w802) -> ()  [unwired: 8 in, 2 out]
          n315 = call "CTRE_Phoenix_MotorControl_SetSelectedSensorPosition.vi"("New Sensor Position"=0, "PhoenixMotorControlDevRef"=w803) -> ()  [unwired: 8 in, 2 out]
          n316 = call "CTRE_Phoenix_MotorControl_Set.vi"("Output"=w804, "Control Mode"=w806, "PhoenixMotorControlDevRef"=w802) -> ()  [unwired: 7 in, 2 out]
          n317 = call "CTRE_Phoenix_MotorControl_Set.vi"("Output"=w804, "Control Mode"=w805, "PhoenixMotorControlDevRef"=w803) -> ()  [unwired: 7 in, 2 out]
        }
        frame #3 {
          n318 = while {
            tunnel: [w816] -> w808
            stop <- w812 stop-if-true
            n319 = call <vilib>:"WPI_DriverStationGame Specific Data.vi"() -> ("Game Specific Data"=w816:string)  [unwired: 11 in]
            n320 = call "Elapsed Time8"("Time Target (s)"=2.0) -> ("Time has Elapsed"=w813:bool)  [unwired: 11 in, 7 out]
            n321 = String Length(string=w816) -> (length=w818:i32)
            n322 = Greater?(x=w818, y=0) -> (0:w814:bool)
            n323 = Or(x=w814, y=w813) -> (x .or. y?=w812:bool)
          }
        }
        frame #4 {
          n324 = String Subset(string=w825, offset (0)=0, length (rest)=1 ("length (rest)")) -> (substring=w824:string)
          n325 = Wait (ms)(milliseconds to wait=u32 500) -> ()  [unwired: 1 out]
          n326 = Equal?(x=w824, y="L") -> (x = y?=w822:bool)
          n327 = Select(t=-1.0, s=w822, f=1.0) -> (s? t:f=w821:dbl)
        }
        frame #5 {
          n328 = while {
            tunnel: w838 -> [w851]
            tunnel: w837 -> [w848]
            tunnel: w836 -> [w849]
            tunnel: [w847] -> w835
            tunnel: [w846] -> w834
            tunnel: [w845] -> w833
            tunnel: w832 -> [w840]
            stop <- w842 stop-if-true
            n329 = local read "angle PID"() -> (w850:T2)
            n330 = Multiply(x=90.0 ("setpoint"), y=w840) -> (x*y=w839:dbl)
            n331 = call "RotateToAngle.vi"("setpoint"=w839, "PID gains"=w850, "PhoenixMotorControlDevRef 2"=w848, "PhoenixMotorControlDevRef"=w849, "navX Device"=w851) -> ("abs(x)"=w844:dbl, "PhoenixMotorControlDevRef 3"=w847:T7, "PhoenixMotorControlDevRef 4"=w846:T7, "navX Device 2"=w845:T14)  [unwired: 3 in]
            n332 = Less?(x=w844, y=5.0) -> (x < y?=w842:bool)
          }
        }
        frame #6 {
          n333 = call "Z900_navX_Set_ZeroYaw.vi"("navX Device"=w856) -> ()  [unwired: 9 in, 2 out]
          n334 = call "CTRE_Phoenix_MotorControl_SetSelectedSensorPosition.vi"("New Sensor Position"=0, "PhoenixMotorControlDevRef"=w852) -> ()  [unwired: 8 in, 2 out]
          n335 = call "CTRE_Phoenix_MotorControl_SetSelectedSensorPosition.vi"("New Sensor Position"=0, "PhoenixMotorControlDevRef"=w853) -> ()  [unwired: 8 in, 2 out]
        }
        frame #7 {
          n336 = while {
            tunnel: w864 -> [w866]
            tunnel: w863 -> [w867]
            tunnel: w862 -> [w865]
            tunnel: [w867] -> w861
            tunnel: [w866] -> w860
            tunnel: [w865] -> w859
            stop <- w871 stop-if-true
            n337 = local read "forward PID"() -> (w875:T2)
            n338 = local read "angle PID"() -> (w876:T2)
            n339 = call "GoDistance.vi"("Forward PID"=w875, "Angle PID"=w876, "x"=4.0, "PhoenixMotorControlDevRef"=w867, "PhoenixMotorControlDevRef 2"=w866, "navX Device"=w865) -> ("Error 2"=w868:dbl, "Error 1"=w870:dbl)  [unwired: 4 in]
            n340 = Less?(x=w868, y=4.0) -> (x < y?=w872:bool)
            n341 = Less?(x=w870, y=60.0) -> (x < y?=w873:bool)
            n342 = And(x=w873, y=w872) -> (x .and. y?=w871:bool)
          }
        }
        frame #8 {
          w883 = 0.0 ("Output")
          w884 = T16 0 items=["PercentOutput"=0, "Position"=1, "Velocity"=2, "Current"=3, "Follower"=5, "MotionProfile"=6, "MotionMagic"=7, "MotionMagicArc"=8, "MotionProfileArc"=10, "Disabled"=15] ("Control Mode")
          w885 = T16 0 items=["PercentOutput"=0, "Position"=1, "Velocity"=2, "Current"=3, "Follower"=5, "MotionProfile"=6, "MotionMagic"=7, "MotionMagicArc"=8, "MotionProfileArc"=10, "Disabled"=15] ("Control Mode")
          n343 = Wait (ms)(milliseconds to wait=u32 500) -> ()  [unwired: 1 out]
          n344 = call "CTRE_Phoenix_MotorControl_SetSelectedSensorPosition.vi"("New Sensor Position"=0, "PhoenixMotorControlDevRef"=w880) -> ()  [unwired: 8 in, 2 out]
          n345 = call "CTRE_Phoenix_MotorControl_SetSelectedSensorPosition.vi"("New Sensor Position"=0, "PhoenixMotorControlDevRef"=w879) -> ()  [unwired: 8 in, 2 out]
          n346 = call "CTRE_Phoenix_MotorControl_Set.vi"("Output"=w883, "Control Mode"=w885, "PhoenixMotorControlDevRef"=w880) -> ()  [unwired: 7 in, 2 out]
          n347 = call "CTRE_Phoenix_MotorControl_Set.vi"("Output"=w883, "Control Mode"=w884, "PhoenixMotorControlDevRef"=w879) -> ()  [unwired: 7 in, 2 out]
        }
        frame #9 {
          n348 = while {
            tunnel: w894 -> [w907]
            tunnel: w893 -> [w906]
            tunnel: w892 -> [w905]
            tunnel: [w900] -> w891
            tunnel: [w899] -> w890
            tunnel: [w898] -> w889
            tunnel: w888 -> [w895]
            stop <- w901 stop-if-true
            n349 = local read "angle PID"() -> (w904:T2)
            n350 = Multiply(x=-90.0 ("setpoint"), y=w895) -> (x*y=w896:dbl)
            n351 = call "RotateToAngle.vi"("setpoint"=w896, "PID gains"=w904, "PhoenixMotorControlDevRef 2"=w906, "PhoenixMotorControlDevRef"=w907, "navX Device"=w905) -> ("abs(x)"=w902:dbl, "PhoenixMotorControlDevRef 3"=w899:T7, "PhoenixMotorControlDevRef 4"=w900:T7, "navX Device 2"=w898:T14)  [unwired: 3 in]
            n352 = Less?(x=w902, y=5.0) -> (x < y?=w901:bool)
          }
        }
        frame #10 {
          n353 = call "Z900_navX_Set_ZeroYaw.vi"("navX Device"=w909) -> ("navX Device"=w908:T14)  [unwired: 9 in, 1 out]
          n354 = call "CTRE_Phoenix_MotorControl_SetSelectedSensorPosition.vi"("New Sensor Position"=0, "PhoenixMotorControlDevRef"=w913) -> ()  [unwired: 8 in, 2 out]
          n355 = call "CTRE_Phoenix_MotorControl_SetSelectedSensorPosition.vi"("New Sensor Position"=0, "PhoenixMotorControlDevRef"=w912) -> ()  [unwired: 8 in, 2 out]
        }
        frame #11 {
          w918 = T16 0 items=["PercentOutput"=0, "Position"=1, "Velocity"=2, "Current"=3, "Follower"=5, "MotionProfile"=6, "MotionMagic"=7, "MotionMagicArc"=8, "MotionProfileArc"=10, "Disabled"=15] ("Control Mode")
          w917 = 0.0 ("Output")
          n356 = call "CTRE_Phoenix_MotorControl_Set.vi"("Output"=w917, "Control Mode"=w918, "PhoenixMotorControlDevRef"=w919) -> ("PhoenixMotorControlDevRef"=w914:T7)  [unwired: 7 in, 1 out]
          n357 = call "CTRE_Phoenix_MotorControl_Set.vi"("Output"=w917, "Control Mode"=w918, "PhoenixMotorControlDevRef"=w920) -> ("PhoenixMotorControlDevRef"=w915:T7)  [unwired: 7 in, 1 out]
        }
        frame #12 {
          n358 = while {
            tunnel: w924 -> [w944]
            tunnel: w923 -> [w943]
            tunnel: w922 -> [w942]
            tunnel: [w927] -> w921
            stop <- w931 stop-if-true
            n359 = local read "angle PID"() -> (w940:T2)
            n360 = local read "forward PID"() -> (w939:T2)
            n361 = call "Elapsed Time9"() -> ("Time has Elapsed"=w932:bool)  [unwired: 12 in, 7 out]
            n362 = call "GoDistanceFast.vi"("Forward PID"=w939, "Angle PID"=w940, "x"=10.0, "PhoenixMotorControlDevRef"=w943, "PhoenixMotorControlDevRef 2"=w942, "navX Device"=w944) -> ("Error 2"=w938:dbl, "Error 1"=w930:dbl)  [unwired: 4 in]
            n363 = Less?(x=w930, y=60.0) -> (x < y?=w935:bool)
            n364 = Less?(x=w938, y=4.0) -> (x < y?=w934:bool)
            n365 = call "CTRE_Phoenix_MotorControl_RefNumRegistryGet.vi"("refnum name"="Elevator") -> ("PhoenixMotorControlDevRef"=w926:T7)  [unwired: 9 in, 1 out]
            n366 = And(x=w935, y=w934) -> (x .and. y?=w933:bool)
            n367 = Less?(x=w930, y=2000.0) -> (x < y?=w928:bool)
            n368 = Or(x=w933, y=w932) -> (x .or. y?=w931:bool)
            n369 = case shown="True" w928 {
              tunnel: [w945 w947] -> w927
              tunnel: w926 -> [w945 w946]
              frame False {
              }
              frame True {
                w948 = T16 0 items=["PercentOutput"=0, "Position"=1, "Velocity"=2, "Current"=3, "Follower"=5, "MotionProfile"=6, "MotionMagic"=7, "MotionMagicArc"=8, "MotionProfileArc"=10, "Disabled"=15] ("Control Mode")
                n370 = call "CTRE_Phoenix_MotorControl_Set.vi"("Output"=1.0, "Control Mode"=w948, "PhoenixMotorControlDevRef"=w946) -> ("PhoenixMotorControlDevRef"=w947:T7)  [unwired: 7 in, 1 out]
              }
            }
          }
        }
        frame #13 {
          n371 = Wait (ms)(milliseconds to wait=u32 500) -> ()  [unwired: 1 out]
        }
        frame #14 {
          w956 = T16 0 items=["PercentOutput"=0, "Position"=1, "Velocity"=2, "Current"=3, "Follower"=5, "MotionProfile"=6, "MotionMagic"=7, "MotionMagicArc"=8, "MotionProfileArc"=10, "Disabled"=15] ("Control Mode")
          n372 = call "CTRE_Phoenix_MotorControl_SetSelectedSensorPosition.vi"("New Sensor Position"=0, "PhoenixMotorControlDevRef"=w952) -> ("PhoenixMotorControlDevRef"=w954:T7)  [unwired: 8 in, 1 out]
          n373 = call "CTRE_Phoenix_MotorControl_Set.vi"("Output"=-1.0, "Control Mode"=w956, "PhoenixMotorControlDevRef"=w954) -> ()  [unwired: 7 in, 2 out]
        }
      }
    }
    frame "Straight" {
      n374 = call "Z900_navX_Set_ZeroYaw.vi"("navX Device"=w958) -> ("navX Device"=w957:T14)  [unwired: 9 in, 1 out]
      n375 = while {
        tunnel: w957 -> [w973]
        tunnel: w960 -> [w972]
        tunnel: w959 -> [w971]
        stop <- w962 stop-if-true
        n376 = local read "forward PID"() -> (w970:T2)
        n377 = local read "angle PID"() -> (w969:T2)
        n378 = call "GoDistance.vi"("Forward PID"=w970, "Angle PID"=w969, "x"=12.0, "PhoenixMotorControlDevRef"=w972, "PhoenixMotorControlDevRef 2"=w971, "navX Device"=w973) -> ("Error 2"=w966:dbl, "Error 1"=w967:dbl)  [unwired: 4 in]
        n379 = Less?(x=w967, y=60.0) -> (x < y?=w964:bool)
        n380 = Less?(x=w966, y=4.0) -> (x < y?=w963:bool)
        n381 = And(x=w964, y=w963) -> (x .and. y?=w962:bool)
      }
    }
    frame "Left" {
      n382 = call <vilib>:"WPI_DriverStationGame Specific Data.vi"() -> ("Game Specific Data"=w982:string)  [unwired: 11 in]
      n383 = String Subset(string=w982, offset (0)=0, length (rest)=1 ("length (rest)")) -> (substring=w979:string)
      n384 = Equal?(x=w979, y="L") -> (x = y?=w977:bool)
      n385 = case shown="True" w977 {
        tunnel: w976 -> [_ w988]
        tunnel: w975 -> [_ w987]
        tunnel: w974 -> [_ w986]
        frame False {
        }
        frame True {
          n386 = flat-sequence {
            tunnel: w988 -> [w994]
            tunnel: w987 -> [w993]
            tunnel: w986 -> [w992]
            tunnel: [w991] -> w985
            tunnel: [w990] -> w984
            tunnel: [w989] -> w983
            tunnel: w985 -> [w1013]
            tunnel: w984 -> [w1012]
            tunnel: w983 -> [w1011]
            frame #0 {
              n387 = while {
                tunnel: w994 -> [w997]
                tunnel: w992 -> [w996]
                tunnel: w993 -> [w995]
                tunnel: [w997] -> w991
                tunnel: [w996] -> w990
                tunnel: [w995] -> w989
                stop <- w999 stop-if-true
                n388 = local read "forward PID"() -> (w1010:T2)
                n389 = local read "angle PID"() -> (w1009:T2)
                n390 = call "GoDistance.vi"("Forward PID"=w1010, "Angle PID"=w1009, "x"=10.0, "PhoenixMotorControlDevRef"=w996, "PhoenixMotorControlDevRef 2"=w995, "navX Device"=w997) -> ("Error 2"=w1006:dbl, "Error 1"=w1007:dbl)  [unwired: 4 in]
                n391 = Less?(x=w1007, y=60.0) -> (x < y?=w1004:bool)
                n392 = Less?(x=w1006, y=4.0) -> (x < y?=w1003:bool)
                n393 = And(x=w1004, y=w1003) -> (x .and. y?=w1001:bool)
                n394 = call "Elapsed Time6"("Time Target (s)"=3.0) -> ("Time has Elapsed"=w1000:bool)  [unwired: 11 in, 7 out]
                n395 = Or(x=w1000, y=w1001) -> (x .or. y?=w999:bool)
              }
            }
            frame #1 {
              n396 = call <vilib>:"WPI_DriverStationGame Specific Data.vi"() -> ("Game Specific Data"=w1019:string)  [unwired: 11 in]
              n397 = String Subset(string=w1019, offset (0)=0, length (rest)=1 ("length (rest)")) -> (substring=w1016:string)
              n398 = Equal?(x=w1016, y="L") -> (x = y?=w1014:bool)
              n399 = case shown="True" w1014 {
                tunnel: w1013 -> [_ w1025]
                tunnel: w1012 -> [_ w1024]
                tunnel: w1011 -> [_ w1023]
                frame False {
                }
                frame True {
                  n400 = flat-sequence {
                    tunnel: w1025 -> [w1031]
                    tunnel: w1024 -> [w1030]
                    tunnel: w1023 -> [w1029]
                    tunnel: [w1028] -> w1022
                    tunnel: [w1027] -> w1021
                    tunnel: [w1026] -> w1020
                    tunnel: w1022 -> [w1045]
                    tunnel: w1021 -> [w1044]
                    tunnel: w1020 -> [w1043]
                    frame #0 {
                      n401 = while {
                        tunnel: w1031 -> [w1042]
                        tunnel: w1030 -> [w1041]
                        tunnel: w1029 -> [w1040]
                        tunnel: [w1034] -> w1028
                        tunnel: [w1033] -> w1027
                        tunnel: [w1032] -> w1026
                        stop <- w1035 stop-if-true
                        n402 = local read "angle PID"() -> (w1039:T2)
                        n403 = call "RotateToAngle.vi"("setpoint"=-90.0, "PID gains"=w1039, "PhoenixMotorControlDevRef 2"=w1040, "PhoenixMotorControlDevRef"=w1041, "navX Device"=w1042) -> ("abs(x)"=w1037:dbl, "PhoenixMotorControlDevRef 3"=w1032:T7, "PhoenixMotorControlDevRef 4"=w1033:T7, "navX Device 2"=w1034:T14)  [unwired: 3 in]
                        n404 = Less?(x=w1037, y=3.0) -> (x < y?=w1035:bool)
                      }
                    }
                    frame #1 {
                      n405 = while {
                        tunnel: w1045 -> [w1061]
                        tunnel: w1044 -> [w1060]
                        tunnel: w1043 -> [w1059]
                        stop <- w1046 stop-if-true
                        n406 = local read "forward PID"() -> (w1057:T2)
                        n407 = local read "angle PID"() -> (w1058:T2)
                        n408 = call "Elapsed Time5"("Time Target (s)"=2.0) -> ("Time has Elapsed"=w1047:bool)  [unwired: 11 in, 7 out]
                        n409 = call "GoDistance.vi"("Forward PID"=w1057, "Angle PID"=w1058, "x"=3.0, "PhoenixMotorControlDevRef"=w1060, "PhoenixMotorControlDevRef 2"=w1059, "navX Device"=w1061) -> ("Error 2"=w1052:dbl, "Error 1"=w1054:dbl)  [unwired: 4 in]
                        n410 = Less?(x=w1054, y=60.0) -> (x < y?=w1050:bool)
                        n411 = Less?(x=w1052, y=3.0) -> (x < y?=w1049:bool)
                        n412 = And(x=w1050, y=w1049) -> (x .and. y?=w1048:bool)
                        n413 = Or(x=w1048, y=w1047) -> (x .or. y?=w1046:bool)
                      }
                    }
                    frame #2 {
                      n414 = while {
                        stop <- w1067 stop-if-true
                        w1065 = T16 0 items=["PercentOutput"=0, "Position"=1, "Velocity"=2, "Current"=3, "Follower"=5, "MotionProfile"=6, "MotionMagic"=7, "MotionMagicArc"=8, "MotionProfileArc"=10, "Disabled"=15] ("Control Mode")
                        n415 = call "CTRE_Phoenix_MotorControl_RefNumRegistryGet.vi"("refnum name"="Elevator") -> ("PhoenixMotorControlDevRef"=w1062:T7)  [unwired: 9 in, 1 out]
                        n416 = call "Elapsed Time14"("Time Target (s)"=0.3) -> ("Time has Elapsed"=w1067:bool)  [unwired: 11 in, 7 out]
                        n417 = call "CTRE_Phoenix_MotorControl_Set.vi"("Output"=0.5, "Control Mode"=w1065, "PhoenixMotorControlDevRef"=w1062) -> ()  [unwired: 7 in, 2 out]
                      }
                    }
                  }
                }
              }
            }
          }
        }
      }
    }
    frame "Right" {
      n418 = call <vilib>:"WPI_DriverStationGame Specific Data.vi"() -> ("Game Specific Data"=w1076:string)  [unwired: 11 in]
      n419 = String Subset(string=w1076, offset (0)=0, length (rest)=1 ("length (rest)")) -> (substring=w1073:string)
      n420 = Equal?(x=w1073, y="L") -> (x = y?=w1071:bool)
      n421 = case shown="True" w1071 {
        tunnel: w1070 -> [_ w1082]
        tunnel: w1069 -> [_ w1081]
        tunnel: w1068 -> [_ w1080]
        frame False {
        }
        frame True {
          n422 = flat-sequence {
            tunnel: w1082 -> [w1088]
            tunnel: w1081 -> [w1087]
            tunnel: w1080 -> [w1086]
            tunnel: [w1085] -> w1079
            tunnel: [w1084] -> w1078
            tunnel: [w1083] -> w1077
            tunnel: w1079 -> [w1107]
            tunnel: w1078 -> [w1106]
            tunnel: w1077 -> [w1105]
            frame #0 {
              n423 = while {
                tunnel: w1088 -> [w1091]
                tunnel: w1086 -> [w1090]
                tunnel: w1087 -> [w1089]
                tunnel: [w1091] -> w1085
                tunnel: [w1090] -> w1084
                tunnel: [w1089] -> w1083
                stop <- w1093 stop-if-true
                n424 = local read "forward PID"() -> (w1104:T2)
                n425 = local read "angle PID"() -> (w1103:T2)
                n426 = call "GoDistance.vi"("Forward PID"=w1104, "Angle PID"=w1103, "x"=10.0, "PhoenixMotorControlDevRef"=w1090, "PhoenixMotorControlDevRef 2"=w1089, "navX Device"=w1091) -> ("Error 2"=w1100:dbl, "Error 1"=w1101:dbl)  [unwired: 4 in]
                n427 = Less?(x=w1101, y=60.0) -> (x < y?=w1098:bool)
                n428 = Less?(x=w1100, y=4.0) -> (x < y?=w1097:bool)
                n429 = And(x=w1098, y=w1097) -> (x .and. y?=w1095:bool)
                n430 = call "Elapsed Time15"("Time Target (s)"=3.0) -> ("Time has Elapsed"=w1094:bool)  [unwired: 11 in, 7 out]
                n431 = Or(x=w1094, y=w1095) -> (x .or. y?=w1093:bool)
              }
            }
            frame #1 {
              n432 = call <vilib>:"WPI_DriverStationGame Specific Data.vi"() -> ("Game Specific Data"=w1113:string)  [unwired: 11 in]
              n433 = String Subset(string=w1113, offset (0)=0, length (rest)=1 ("length (rest)")) -> (substring=w1110:string)
              n434 = Equal?(x=w1110, y="R") -> (x = y?=w1108:bool)
              n435 = case shown="True" w1108 {
                tunnel: w1107 -> [_ w1119]
                tunnel: w1106 -> [_ w1118]
                tunnel: w1105 -> [_ w1117]
                frame False {
                }
                frame True {
                  n436 = flat-sequence {
                    tunnel: w1119 -> [w1125]
                    tunnel: w1118 -> [w1124]
                    tunnel: w1117 -> [w1123]
                    tunnel: [w1122] -> w1116
                    tunnel: [w1121] -> w1115
                    tunnel: [w1120] -> w1114
                    tunnel: w1116 -> [w1139]
                    tunnel: w1115 -> [w1138]
                    tunnel: w1114 -> [w1137]
                    frame #0 {
                      n437 = while {
                        tunnel: w1125 -> [w1136]
                        tunnel: w1124 -> [w1135]
                        tunnel: w1123 -> [w1134]
                        tunnel: [w1128] -> w1122
                        tunnel: [w1127] -> w1121
                        tunnel: [w1126] -> w1120
                        stop <- w1129 stop-if-true
                        n438 = local read "angle PID"() -> (w1133:T2)
                        n439 = call "RotateToAngle.vi"("setpoint"=90.0, "PID gains"=w1133, "PhoenixMotorControlDevRef 2"=w1134, "PhoenixMotorControlDevRef"=w1135, "navX Device"=w1136) -> ("abs(x)"=w1131:dbl, "PhoenixMotorControlDevRef 3"=w1126:T7, "PhoenixMotorControlDevRef 4"=w1127:T7, "navX Device 2"=w1128:T14)  [unwired: 3 in]
                        n440 = Less?(x=w1131, y=3.0) -> (x < y?=w1129:bool)
                      }
                    }
                    frame #1 {
                      n441 = while {
                        tunnel: w1139 -> [w1155]
                        tunnel: w1138 -> [w1154]
                        tunnel: w1137 -> [w1153]
                        stop <- w1140 stop-if-true
                        n442 = local read "forward PID"() -> (w1151:T2)
                        n443 = local read "angle PID"() -> (w1152:T2)
                        n444 = call "Elapsed Time16"("Time Target (s)"=2.0) -> ("Time has Elapsed"=w1141:bool)  [unwired: 11 in, 7 out]
                        n445 = call "GoDistance.vi"("Forward PID"=w1151, "Angle PID"=w1152, "x"=3.0, "PhoenixMotorControlDevRef"=w1154, "PhoenixMotorControlDevRef 2"=w1153, "navX Device"=w1155) -> ("Error 2"=w1146:dbl, "Error 1"=w1148:dbl)  [unwired: 4 in]
                        n446 = Less?(x=w1148, y=60.0) -> (x < y?=w1144:bool)
                        n447 = Less?(x=w1146, y=3.0) -> (x < y?=w1143:bool)
                        n448 = And(x=w1144, y=w1143) -> (x .and. y?=w1142:bool)
                        n449 = Or(x=w1142, y=w1141) -> (x .or. y?=w1140:bool)
                      }
                    }
                    frame #2 {
                      n450 = while {
                        stop <- w1161 stop-if-true
                        w1159 = T16 0 items=["PercentOutput"=0, "Position"=1, "Velocity"=2, "Current"=3, "Follower"=5, "MotionProfile"=6, "MotionMagic"=7, "MotionMagicArc"=8, "MotionProfileArc"=10, "Disabled"=15] ("Control Mode")
                        n451 = call "CTRE_Phoenix_MotorControl_RefNumRegistryGet.vi"("refnum name"="Elevator") -> ("PhoenixMotorControlDevRef"=w1156:T7)  [unwired: 9 in, 1 out]
                        n452 = call "Elapsed Time17"("Time Target (s)"=0.3) -> ("Time has Elapsed"=w1161:bool)  [unwired: 11 in, 7 out]
                        n453 = call "CTRE_Phoenix_MotorControl_Set.vi"("Output"=0.5, "Control Mode"=w1159, "PhoenixMotorControlDevRef"=w1156) -> ()  [unwired: 7 in, 2 out]
                      }
                    }
                  }
                }
              }
            }
          }
        }
      }
    }
    frame "Stop" {
    }
  }
